vi "nano MALDI spotter v1.2.vi"() -> ()   [LabVIEW 2014]
uses:
  <vilib>/MakerHub/LINX/Public/Peripherals/Digital/Digital Write 1 Chan.vi
  <vilib>/MakerHub/LINX/Public/Peripherals/Digital/Digital Read 1 Chan.vi
  <vilib>/MakerHub/LINX/Public/Peripherals/Digital/Digital Write N Chans.vi
  <vilib>/MakerHub/LINX/Public/Peripherals/Digital/Digital Read N Chans.vi
  <vilib>/MakerHub/LINX/Private/Local IO/LinxDigitalWrite.vi
  <vilib>/MakerHub/LINX/Public/Utilities/Check Channel.vi
  <vilib>/MakerHub/LINX/Private/Local IO/LinxDigitalRead.vi
  <vilib>/MakerHub/LINX/Public/Utilities/Open Serial.vi
  <vilib>/MakerHub/LINX/Private/Utilties/Generate Error.vi
  <vilib>/MakerHub/LINX/LMH-LINX.lvlib
panel:
  out "number of spots":i8
  out "R of B/49":dbl
  out "IQ of B/49":dbl
  out "B-25":dbl
  out "First point(row)=Last point(row) ?":bool
  out "B\n=Number of spots except the first row":dbl
  out "B-1\n= # of spots in the last row\n= (# of spots - first row -1)":dbl
  out "IQ of B/25 = 0":bool
  out "IQ of B/49 = 0":bool
  out "A\n= 24-start point(column)+1\n= # of spots in the first row":dbl
  out "24-start point(columm)":dbl
  out "Last point(column)-Start point(column)":dbl
  out "milliseconds to wait 2":u32
  in  "stop":bool
  in  "Tab Control":T1(tab)=enum."Motor control"
  in  "Loop Control":bool=TRUE
  in  "Serial Port":refnum<visa-resource-name>="COM8" caption="Serial Port 2"
  in  "Digital Output Channel Channel":u8=13
  in  "LED Control":bool
  in  "OPTIONS":enum16{"OFF", "syringe", "X axis", "Y axis"}(ring)
  in  "*  Light On - Counterclockwise\n*  Light Off - Clockwise":bool
  in  "Value":bool
  in  "Value 2":bool=TRUE
  in  "FREQUENCY (Hz)":u32=50
  in  "Frequency (Hz) 2":u32(slide)=450 scale=50.0..450.0
  in  "Frequency (Hz) 3":u32(slide)=450 scale=50.0..450.0
  in  "MILLISECONDS":u32=40
  in  "SWITCH":bool=TRUE
  in  "Time per spots(s)":i8
  in  "Last point(column)":dbl
  in  "Start point(column)":dbl
  in  "Start point, row":dbl
  in  "Last point, row":dbl
  in  "RUN":bool
  in  "Total elution time\n(min)":sgl
  # "Nano-LC MALDI Spotter Robot"
  # "Instructions:\n1.Set Arduino Serial port.\n2.Choose the default LED DO channel(13). \n3.Confirm that LED control operates normally."
  # "Instructions:\n1.Change the options before operating motors\n2.Turn on the light to rotate moter counterclockwise.\n3.To speed up the motor speed, increase the FREQEUNCY and decrease MILLISECONDS.\n4.Before changing to another tab, click stop button."
  # "Instructions:\nTo start autohome, click SWITCH"
  # "Instructions:\n1. Fill in the blank. Refer to the picture below\n2. You can choose whether matrix motor will be operated or not\n3. Click RUN to start spotting"
  # "Please insert corresponding number in  \"Row\" blank box.\nA=1, B=2, C=3, D=4, E=5, F=6, G=7, H=8, I=9, J=10, K=11, \nL= 12, M=13, N=14, O=15, P=16"
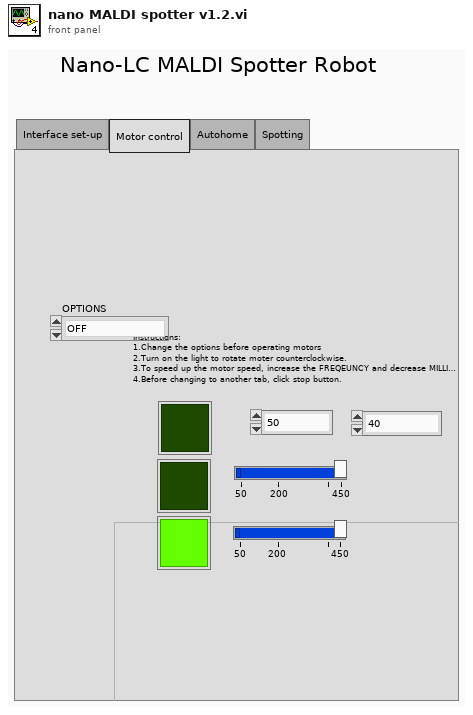
[diagram p1: front panel]
types:
  T1 = enum32{"Interface set-up", "Motor control", "Autohome", "Spotting"}
  T2 = typedef "LMH-LINX.lvlib/LINX Ref.ctl" = cluster{"IO":T3, "Interface":T4, "LINX Device Config":T5}
  T3 = typedef "LMH-LINX.lvlib/Platform.ctl" = enum16{"Remote", "Local"}
  T4 = typedef "LMH-LINX.lvlib/Interface.ctl" = enum16{"Serial", "TCP"}
  T5 = typedef "LMH-LINX.lvlib/Device.lvlib/LINX Device Config.ctl" = cluster{"Interface":T4, "COM Port":refnum<visa-resource-name>, "TCP Configuration":T6, "Device Family":u8, "Device ID":u8, "Device Name":string, "TCP Ref":refnum<k5>, "Channels":T7}
  T6 = typedef "LMH-LINX.lvlib/Device.lvlib/TCP Config.ctl" = cluster{"IP Address":string, "Port":u16}
  T7 = typedef "LMH-LINX.lvlib/Channels.ctl" = cluster{"DI":u8[], "DO":u8[], "AI":u8[], "AO":u8[], "PWM":u8[], "QE":u8[], "UART":u8[], "I2C 2":u8[], "SPI":u8[], "CAN":u8[], "Servo":u8[], "AI Ref (V)":dbl, "AI Resolution (Bits)":u8, "AO Ref (V)":dbl, "AO Resolution (Bits)":u8}
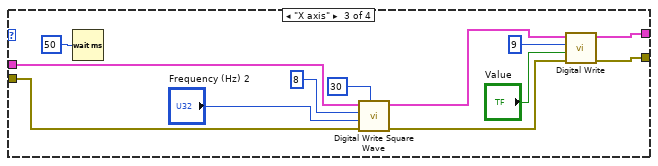
[diagram p5: hidden frame]
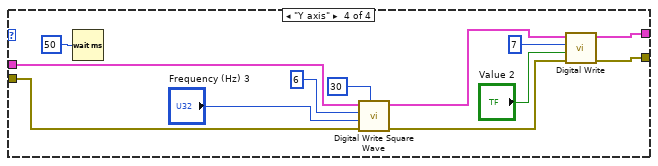
[diagram p6: hidden frame]
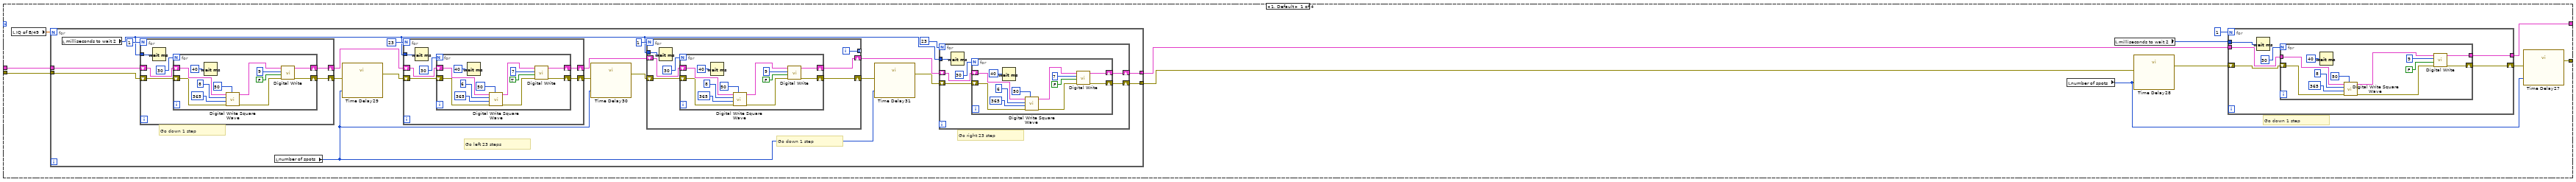
[diagram p10: hidden frame]
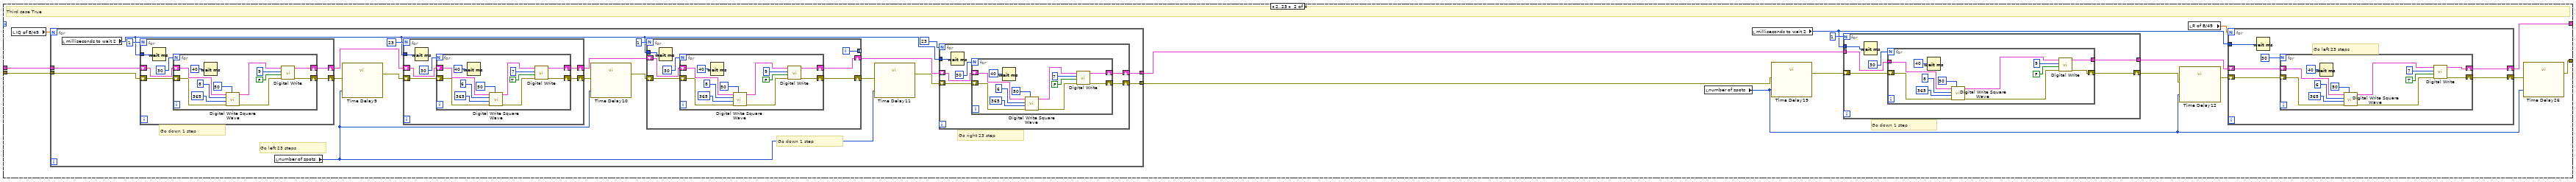
[diagram p11: hidden frame]
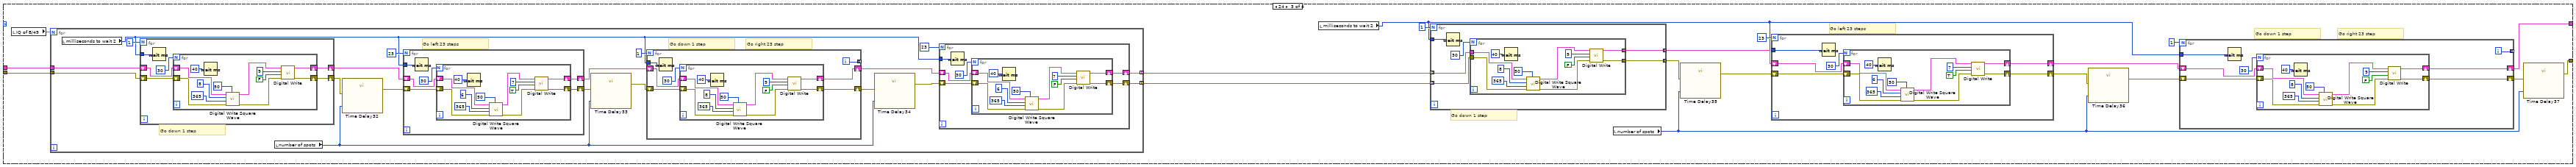
[diagram p12: hidden frame]
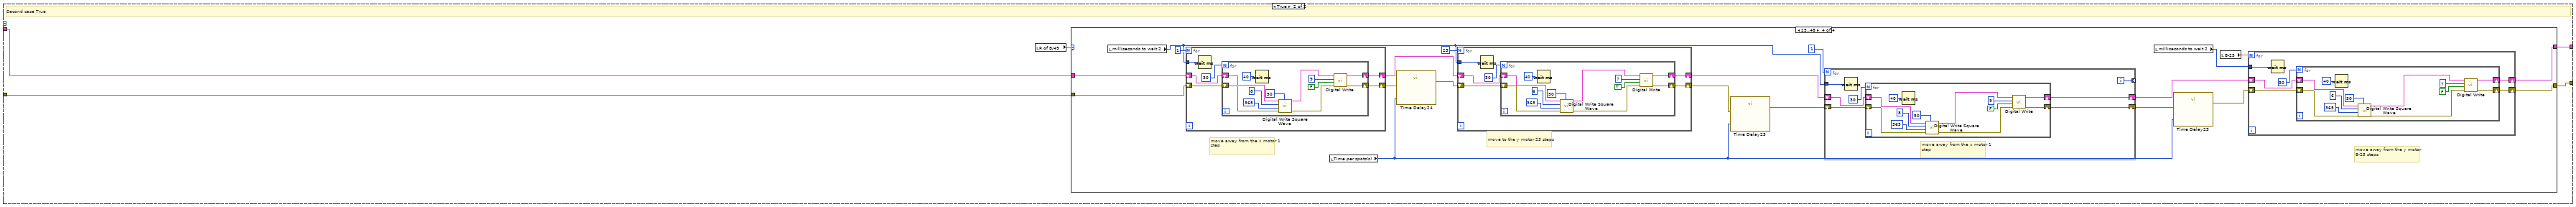
[diagram p13: hidden frame]
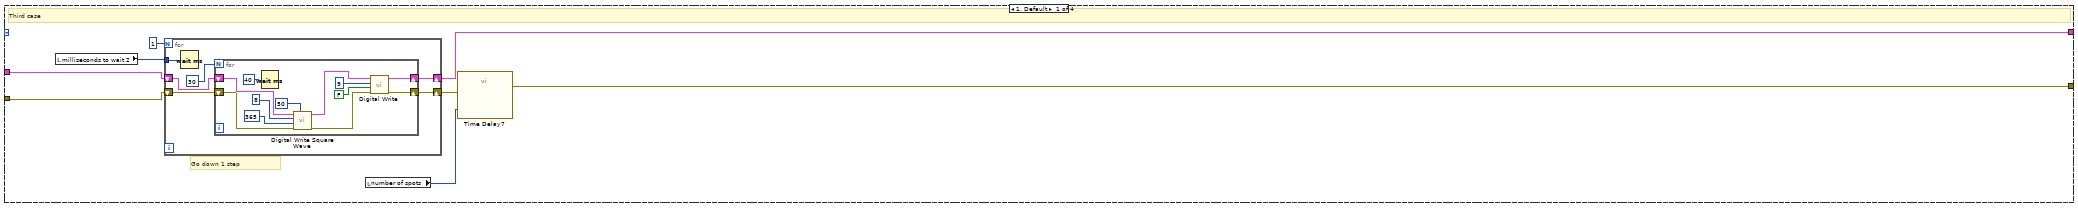
[diagram p14: hidden frame]
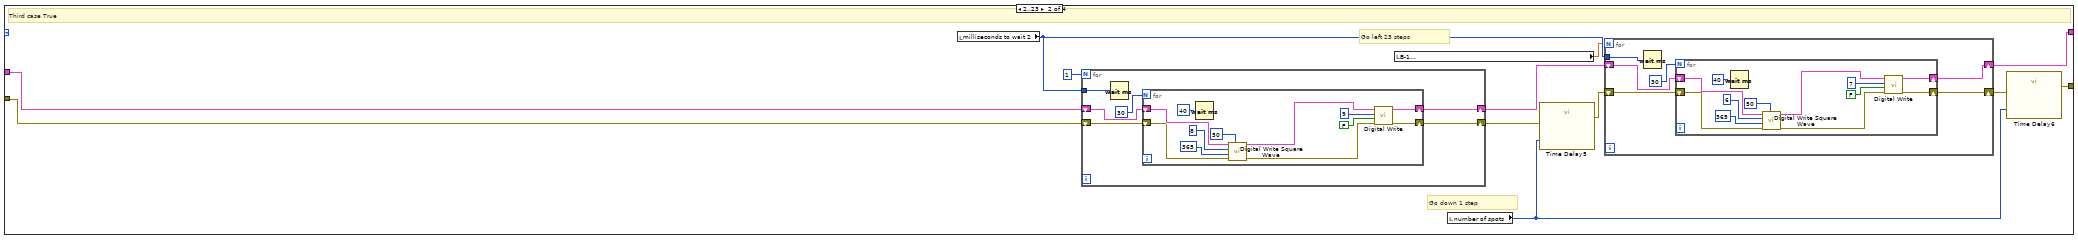
[diagram p15: hidden frame]
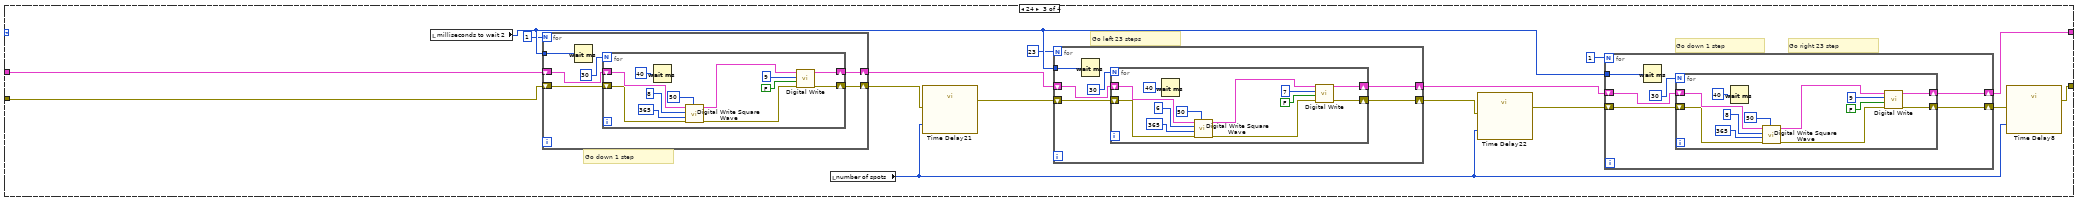
[diagram p16: hidden frame]
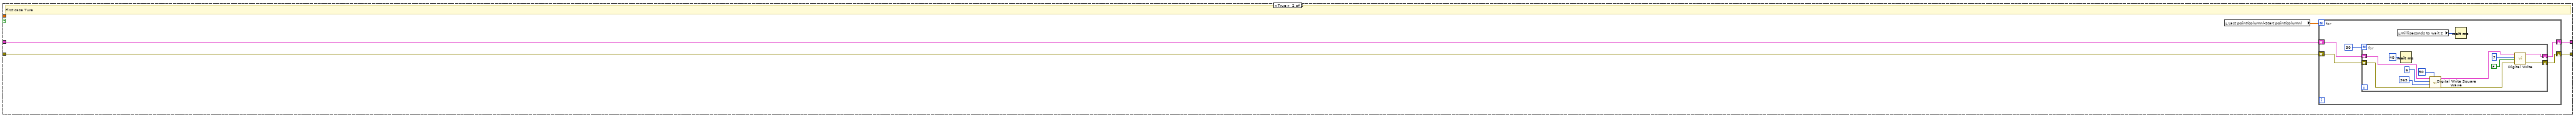
[diagram p17: hidden frame]
diagram:
  # "Option 선택용 Tab control\n-setting\n-autohome\n-motor control\n-spotting"
  # "4."
  n1 = call-poly <vilib>:"Open.vi"("Error In"=errorcluster {"status"=FALSE, "code"=0, "source"=""}, "Serial Port"="Serial Port") -> ("Error Out"=w3:errorcluster, "LINX Resource"=w4:T2)  [unwired: 7 in, 1 out]
  n2 = while {
    tunnel: w4 -> [w12]
    tunnel: w3 -> [w11]
    tunnel: [w10] -> w2
    tunnel: [w9] -> w1
    stop <- "stop" stop-if-true
    n3 = case shown="\"Spotting\"" "Tab Control" {
      tunnel: w12 -> [w17 w30 w71 w205]
      tunnel: w11 -> [w16 w29 w72 w206]
      tunnel: [w15 w28 w70 w180] -> w10
      tunnel: [w14 w27 w69 w179] -> w9
      frame "Interface set-up", Default {
        # "1. Open a connection to the LINX device.\n3. Write the value to the specified DO channel.\n4. Close the connection to the LINX device.\n5. Handle Errors"
        # "LED control\nIf it is well operated, labview and arduino is connected."
        n4 = while {
          tunnel: w17 -> [w24]
          tunnel: [w23] -> w15
          shift-right: [w21] -> w14
          shift-left: w16 -> [w22]
          stop <- w25 stop-if-true
          n5 = call-poly <vilib>:"Digital Write.vi"("Error In"=w22, "Output Value"="LED Control", "DO Channel"="Digital Output Channel Channel", "LINX Resource"=w24) -> ("Error Out"=w21:errorcluster, "LINX Resource"=w23:T2)  [unwired: 6 in]
          n6 = Or(x=w21, y="Loop Control") -> (x .or. y?=w25:bool)
        }
      }
      frame "Motor control" {
        n7 = case shown="\"syringe\"" "OPTIONS" {
          tunnel: w30 -> [w32 w44 w54 w68]
          tunnel: w29 -> [w31 w43 w53 w67]
          tunnel: [w32 w42 w56 w66] -> w28
          tunnel: [w31 w41 w55 w65] -> w27
          frame "OFF", Default {
          }
          frame "syringe" {
            # "Syringe motor On/Off\n-True=On\n-False=Off, 다른 option 대기"
            n8 = Wait (ms)(milliseconds to wait="MILLISECONDS") -> ()  [unwired: 1 out]
            n9 = call <vilib>:"Digital Write Square Wave.vi"("Duration (ms)"=u32 50, "Error In"=w43, "Frequency (Hz)"="FREQUENCY (Hz)", "Channel"=u8 10, "LINX Resource"=w44) -> ("Error Out"=w39:errorcluster, "LINX Resource"=w40:T2)  [unwired: 5 in]
            n10 = call-poly <vilib>:"Digital Write.vi"("Error In"=w39, "Output Value"="*  Light On - Counterclockwise\n*  Light Off - Clockwise", "DO Channel"=u8 11, "LINX Resource"=w40) -> ("Error Out"=w41:errorcluster, "LINX Resource"=w42:T2)  [unwired: 6 in]
          }
          frame "X axis" {
            n11 = Wait (ms)(milliseconds to wait=u32 50) -> ()  [unwired: 1 out]
            n12 = call <vilib>:"Digital Write Square Wave.vi"("Duration (ms)"=u32 30, "Error In"=w53, "Frequency (Hz)"="Frequency (Hz) 2", "Channel"=u8 8, "LINX Resource"=w54) -> ("Error Out"=w51:errorcluster, "LINX Resource"=w52:T2)  [unwired: 5 in]
            n13 = call-poly <vilib>:"Digital Write.vi"("Error In"=w51, "Output Value"="Value", "DO Channel"=u8 9, "LINX Resource"=w52) -> ("Error Out"=w55:errorcluster, "LINX Resource"=w56:T2)  [unwired: 6 in]
          }
          frame "Y axis" {
            n14 = Wait (ms)(milliseconds to wait=u32 50) -> ()  [unwired: 1 out]
            n15 = call <vilib>:"Digital Write Square Wave.vi"("Duration (ms)"=u32 30, "Error In"=w67, "Frequency (Hz)"="Frequency (Hz) 3", "Channel"=u8 6, "LINX Resource"=w68) -> ("Error Out"=w63:errorcluster, "LINX Resource"=w64:T2)  [unwired: 5 in]
            n16 = call-poly <vilib>:"Digital Write.vi"("Error In"=w63, "Output Value"="Value 2", "DO Channel"=u8 7, "LINX Resource"=w64) -> ("Error Out"=w65:errorcluster, "LINX Resource"=w66:T2)  [unwired: 6 in]
          }
        }
      }
      frame "Autohome" {
        n17 = event shown="[0] \"SWITCH\": Value Change" {
          selector: _ -> [_]
          dyn-events: _ -> [_]
          timeout: _ -> [_]
          tunnel: w72 -> [w79]
          tunnel: w71 -> [w80]
          tunnel: [w84] -> w70
          tunnel: [w83] -> w69
          event "SWITCH": Value Change {
            # "Autohome option On/Off 컨트롤"
            # "*Y axis autohome\n1) if digital reads #4, motor stops to rotate.\n2) Motor rotates to go to the position of sink."
            # "*X axis autohome\n1) if digital reads #5, motor stops to rotate.\n2) Motor rotates to go to the position of sink."
            n18 = event-data() -> ()  [unwired: 1 in, 6 out]
            n19 = while {
              tunnel: w80 -> [w108]
              tunnel: [w118] -> w78
              tunnel: [w115] -> w77
              tunnel: w79 -> [w107]
              stop <- w114 stop-if-true
              n20 = Wait (ms)(milliseconds to wait=u32 50) -> ()  [unwired: 1 out]
              n21 = call <vilib>:"Digital Write Square Wave.vi"("Duration (ms)"=u32 30, "Error In"=w107, "Frequency (Hz)"=u32 450, "Channel"=u8 8, "LINX Resource"=w108) -> ("Error Out"=w112:errorcluster, "LINX Resource"=w113:T2)  [unwired: 5 in]
              n22 = call-poly <vilib>:"Digital Write.vi"("Error In"=w112, "Output Value"=TRUE, "DO Channel"=u8 9, "LINX Resource"=w113) -> ("Error Out"=w105:errorcluster, "LINX Resource"=w106:T2)  [unwired: 6 in]
              n23 = call-poly <vilib>:"Digital Read.vi"("Error In"=w105, "DI Channel"=u8 5 ("Analog Channel"), "LINX Resource"=w106) -> ("Error Out"=w115:errorcluster, "DI Value"=w116:bool, "LINX Resource"=w118:T2)  [unwired: 6 in]
              n24 = Or(x=w116, y=w115) -> (x .or. y?=w114:bool)
            }
            n25 = for {
              N: 83 -> [_]
              tunnel: w78 -> [w135]
              tunnel: [w133] -> w76
              tunnel: [w132] -> w75
              tunnel: w77 -> [w134]
              n26 = Wait (ms)(milliseconds to wait=u32 50) -> ()  [unwired: 1 out]
              n27 = call <vilib>:"Digital Write Square Wave.vi"("Duration (ms)"=u32 50, "Error In"=w134, "Frequency (Hz)"=u32 400, "Channel"=u8 8, "LINX Resource"=w135) -> ("Error Out"=w141:errorcluster, "LINX Resource"=w142:T2)  [unwired: 5 in]
              n28 = call-poly <vilib>:"Digital Write.vi"("Error In"=w141, "Output Value"=FALSE, "DO Channel"=u8 9, "LINX Resource"=w142) -> ("Error Out"=w132:errorcluster, "LINX Resource"=w133:T2)  [unwired: 6 in]
            }
            n29 = while {
              tunnel: w76 -> [w91]
              tunnel: [w101] -> w74
              tunnel: [w98] -> w73
              tunnel: w75 -> [w90]
              stop <- w97 stop-if-true
              n30 = Wait (ms)(milliseconds to wait=u32 50) -> ()  [unwired: 1 out]
              n31 = call <vilib>:"Digital Write Square Wave.vi"("Duration (ms)"=u32 30, "Error In"=w90, "Frequency (Hz)"=u32 450, "Channel"=u8 6, "LINX Resource"=w91) -> ("Error Out"=w95:errorcluster, "LINX Resource"=w96:T2)  [unwired: 5 in]
              n32 = call-poly <vilib>:"Digital Write.vi"("Error In"=w95, "Output Value"=TRUE, "DO Channel"=u8 7, "LINX Resource"=w96) -> ("Error Out"=w88:errorcluster, "LINX Resource"=w89:T2)  [unwired: 6 in]
              n33 = call-poly <vilib>:"Digital Read.vi"("Error In"=w88, "DI Channel"=u8 4 ("Analog Channel"), "LINX Resource"=w89) -> ("Error Out"=w98:errorcluster, "DI Value"=w99:bool, "LINX Resource"=w101:T2)  [unwired: 6 in]
              n34 = Or(x=w99, y=w98) -> (x .or. y?=w97:bool)
            }
            n35 = for {
              N: 260 -> [_]
              tunnel: [w121] -> w84
              shift-right: [w120] -> w83
              shift-left: w73 -> [w130]
              tunnel: w74 -> [w122]
              n36 = Wait (ms)(milliseconds to wait=u32 50) -> ()  [unwired: 1 out]
              n37 = call <vilib>:"Digital Write Square Wave.vi"("Duration (ms)"=u32 50, "Error In"=w130, "Frequency (Hz)"=u32 400, "Channel"=u8 6, "LINX Resource"=w122) -> ("Error Out"=w128:errorcluster, "LINX Resource"=w129:T2)  [unwired: 5 in]
              n38 = call-poly <vilib>:"Digital Write.vi"("Error In"=w128, "Output Value"=FALSE, "DO Channel"=u8 7, "LINX Resource"=w129) -> ("Error Out"=w120:errorcluster, "LINX Resource"=w121:T2)  [unwired: 6 in]
            }
          }
        }
      }
      frame "Spotting" {
        # "Case 1 : Is it Row of start position=Row of last position?\nTrue : Move just as the value(Column position of last - column position of first)\nFalse :  First, move right just as the value, 24 - Start position(column)"
        # "Setting start position of row from (1,1)\nTrue : Row position of start point - 1 = 0, don't move \nFalse : Riw position of start point -1 is not 0. \n          move downward just as many as the value"
        # "Move from the position of sink to (1,1)"
        # "Setting start position of column from (1,1)\nTrue : Column position of start point - 1 = 0, don't move \nFalse : Column position of start point -1 is not 0. \n          move downward just as many as the value"
        n39 = event shown="[0] \"RUN\": Value Change" {
          selector: _ -> [_]
          dyn-events: _ -> [_]
          timeout: _ -> [_]
          tunnel: [w332] -> w209
          tunnel: [w331] -> w208
          tunnel: w206 -> [w330]
          tunnel: w205 -> [w329]
          event "RUN": Value Change {
            n40 = event-data() -> ()  [unwired: 1 in, 6 out]
            n41 = for {
              N: 130 -> [_]
              tunnel: [w354] -> w326
              shift-right: [w348] -> w325
              shift-left: w330 -> [w356]
              tunnel: w329 -> [w346]
              n42 = Wait (ms)(milliseconds to wait=u32 50) -> ()  [unwired: 1 out]
              n43 = call <vilib>:"Digital Write Square Wave.vi"("Duration (ms)"=u32 50, "Error In"=w356, "Frequency (Hz)"=u32 400, "Channel"=u8 8, "LINX Resource"=w346) -> ("Error Out"=w353:errorcluster, "LINX Resource"=w355:T2)  [unwired: 5 in]
              n44 = call-poly <vilib>:"Digital Write.vi"("Error In"=w353, "Output Value"=FALSE, "DO Channel"=u8 9, "LINX Resource"=w355) -> ("Error Out"=w348:errorcluster, "LINX Resource"=w354:T2)  [unwired: 6 in]
            }
            n45 = call "Time Delay"("error in (no error)"=w325, "Delay Time (s)"=1.0) -> ("error out"=w324:errorcluster)  [unwired: 9 in]
            n46 = for {
              N: 130 -> [_]
              tunnel: [w342] -> w332
              shift-right: [w336] -> w331
              shift-left: w324 -> [w344]
              tunnel: w326 -> [w334]
              n47 = Wait (ms)(milliseconds to wait=u32 50) -> ()  [unwired: 1 out]
              n48 = call <vilib>:"Digital Write Square Wave.vi"("Duration (ms)"=u32 50, "Error In"=w344, "Frequency (Hz)"=u32 400, "Channel"=u8 6, "LINX Resource"=w334) -> ("Error Out"=w341:errorcluster, "LINX Resource"=w343:T2)  [unwired: 5 in]
              n49 = call-poly <vilib>:"Digital Write.vi"("Error In"=w341, "Output Value"=FALSE, "DO Channel"=u8 7, "LINX Resource"=w343) -> ("Error Out"=w336:errorcluster, "LINX Resource"=w342:T2)  [unwired: 6 in]
            }
          }
        }
        n50 = Subtract(x="Last point(column)", y="Start point(column)") -> (x-y=→"Last point(column)-Start point(column)":dbl)
        n51 = Subtract(x="Start point(column)", y=1.0) -> (x-y=w165:dbl)
        n52 = Subtract(x=24.0, y="Start point(column)") -> (x-y=w160:dbl)
        "24-start point(columm)" <- w160
        n53 = Increment(x=w160) -> (x+1=→"A\n= 24-start point(column)+1\n= # of spots in the first row":dbl)
        n54 = Equal?(x=0.0, y=w165) -> (x = y?=w199:bool)
        n55 = case shown="False" w199 {
          tunnel: [w302 w321] -> w211
          tunnel: [w303 w322] -> w210
          tunnel: w209 -> [w301 w322]
          tunnel: w208 -> [w300 w321]
          tunnel: w165 -> [w299 _]
          frame False {
            n56 = for {
              N: w299 -> [_]
              shift-right: [w308] -> w303
              shift-left: w301 -> [w306]
              shift-right: [w307] -> w302
              shift-left: w300 -> [w305]
              n57 = for {
                N: 30 -> [_]
                tunnel: [w318] -> w308
                shift-right: [w312] -> w307
                shift-left: w305 -> [w320]
                tunnel: w306 -> [w309]
                n58 = Wait (ms)(milliseconds to wait=u32 40) -> ()  [unwired: 1 out]
                n59 = call <vilib>:"Digital Write Square Wave.vi"("Duration (ms)"=u32 50, "Error In"=w320, "Frequency (Hz)"=u32 365, "Channel"=u8 8, "LINX Resource"=w309) -> ("Error Out"=w317:errorcluster, "LINX Resource"=w319:T2)  [unwired: 5 in]
                n60 = call-poly <vilib>:"Digital Write.vi"("Error In"=w317, "Output Value"=TRUE, "DO Channel"=u8 9, "LINX Resource"=w319) -> ("Error Out"=w312:errorcluster, "LINX Resource"=w318:T2)  [unwired: 6 in]
              }
            }
          }
          frame True {
          }
        }
        n61 = Subtract(x=24.0, y="Start point, row") -> ()  [unwired: 1 out]
        n62 = Subtract(x="Last point, row", y="Start point, row") -> (x-y=w191:dbl)
        n63 = Subtract(x="Start point, row", y=1.0) -> (x-y=w164:dbl)
        n64 = call "Time Delay2"("error in (no error)"=w211, "Delay Time (s)"=1.0) -> ("error out"=w212:errorcluster)  [unwired: 9 in]
        n65 = Multiply(x=30.0, y=w164) -> ()  [unwired: 1 out]
        n66 = Equal?(x=0.0, y=w191) -> (x = y?=→"First point(row)=Last point(row) ?":bool)
        n67 = Equal?(x=0.0, y=w164) -> (x = y?=w198:bool)
        n68 = case shown="False" w198 {
          tunnel: w212 -> [w278 w297]
          tunnel: w210 -> [w279 w298]
          tunnel: [w277 w298] -> w207
          tunnel: [w276 w297] -> w193
          tunnel: w164 -> [w275 _]
          frame False {
            n69 = for {
              N: w275 -> [_]
              shift-right: [w282] -> w277
              shift-left: w279 -> [w284]
              shift-right: [w281] -> w276
              shift-left: w278 -> [w283]
              n70 = for {
                N: 30 -> [_]
                tunnel: [w294] -> w282
                shift-right: [w288] -> w281
                shift-left: w283 -> [w296]
                tunnel: w284 -> [w286]
                n71 = Wait (ms)(milliseconds to wait=u32 40) -> ()  [unwired: 1 out]
                n72 = call <vilib>:"Digital Write Square Wave.vi"("Duration (ms)"=u32 50, "Error In"=w296, "Frequency (Hz)"=u32 365, "Channel"=u8 6, "LINX Resource"=w286) -> ("Error Out"=w293:errorcluster, "LINX Resource"=w295:T2)  [unwired: 5 in]
                n73 = call-poly <vilib>:"Digital Write.vi"("Error In"=w293, "Output Value"=FALSE, "DO Channel"=u8 7, "LINX Resource"=w295) -> ("Error Out"=w288:errorcluster, "LINX Resource"=w294:T2)  [unwired: 6 in]
              }
            }
          }
          frame True {
            # "subVI\nSetting start position of y"
          }
        }
        n74 = local read "A\n= 24-start point(column)+1\n= # of spots in the first row"() -> (w158:dbl)
        n75 = Multiply(x="Total elution time\n(min)", y=sgl 60.0) -> (x*y=w145:sgl)
        n76 = Divide(x=w145, y="Time per spots(s)") -> (x/y=→"number of spots":sgl)
        n77 = local read "number of spots"() -> (w147:i8)
        n78 = local read "First point(row)=Last point(row) ?"() -> (w152:bool)
        n79 = Subtract(x=w147, y=w158) -> (x-y=w155:dbl)
        "B\n=Number of spots except the first row" <- w155
        n80 = call "Time Delay3"("error in (no error)"=w193, "Delay Time (s)"="Time per spots(s)") -> ("error out"=w192:errorcluster)  [unwired: 9 in]
        n81 = Decrement(x=w155) -> (x-1=→"B-1\n= # of spots in the last row\n= (# of spots - first row -1)":dbl)
        n82 = Multiply(x=u32 1000, y="Time per spots(s)") -> (x*y=→"milliseconds to wait 2":u32)
        n83 = Subtract(x=w155, y=25.0) -> (x-y=w167:dbl)
        n84 = Quotient & Remainder(x=w155, y=49.0) -> (x-y*floor(x/y)=w172:dbl, floor(x/y)=w166:dbl)
        "IQ of B/49" <- w166
        "R of B/49" <- w172
        n85 = case shown="False" w152 {
          tunnel: w192 -> [w366 w1256]
          tunnel: w207 -> [w367 w1257]
          tunnel: [w362 w1254] -> w178
          tunnel: [w361 w1255] -> w177
          tunnel: w167 -> [_ _]
          frame False {
            # "first row"
            # "First case False"
            n86 = local read "24-start point(columm)"() -> (w358:dbl)
            n87 = local read "milliseconds to wait 2"() -> (w359:u32)
            n88 = for {
              N: w358 -> [_]
              shift-right: [w1238] -> w364
              shift-left: w367 -> [w1240]
              shift-right: [w1237] -> w365
              shift-left: w366 -> [w1239]
              tunnel: w359 -> [w1235]
              n89 = Wait (ms)(milliseconds to wait=w1235) -> ()  [unwired: 1 out]
              n90 = for {
                N: 30 -> [_]
                tunnel: [w1250] -> w1238
                shift-right: [w1244] -> w1237
                shift-left: w1239 -> [w1252]
                tunnel: w1240 -> [w1241]
                n91 = Wait (ms)(milliseconds to wait=u32 40) -> ()  [unwired: 1 out]
                n92 = call <vilib>:"Digital Write Square Wave.vi"("Duration (ms)"=u32 50, "Error In"=w1252, "Frequency (Hz)"=u32 365, "Channel"=u8 6, "LINX Resource"=w1241) -> ("Error Out"=w1249:errorcluster, "LINX Resource"=w1251:T2)  [unwired: 5 in]
                n93 = call-poly <vilib>:"Digital Write.vi"("Error In"=w1249, "Output Value"=FALSE, "DO Channel"=u8 7, "LINX Resource"=w1251) -> ("Error Out"=w1244:errorcluster, "LINX Resource"=w1250:T2)  [unwired: 6 in]
              }
            }
            n94 = local read "Time per spots(s)"() -> (w360:i8)
            n95 = local read "IQ of B/49 = 0"() -> (w357:bool)
            n96 = call "Time Delay4"("error in (no error)"=w365, "Delay Time (s)"=w360) -> ("error out"=w363:errorcluster)  [unwired: 9 in]
            n97 = case shown="False" w357 {
              tunnel: w364 -> [w370 w997]
              tunnel: w363 -> [w369 w996]
              tunnel: [w372 w994] -> w362
              tunnel: [w371 w993] -> w361
              frame False {
                # "Second case False"
                n98 = local read "R of B/49"() -> (w368:dbl)
                n99 = case shown="25..48" w368 {
                  tunnel: [w375 w500 w641 w808] -> w372
                  tunnel: [w376 w506 w642 w811] -> w371
                  tunnel: w370 -> [w374 w496 w640 w827]
                  tunnel: w369 -> [w373 w495 w639 w826]
                  frame 1, Default {
                    # "Go down 1 step"
                    n100 = local read "IQ of B/49"() -> (w377:dbl)
                    n101 = for {
                      N: w377 -> [_]
                      tunnel: [w403] -> w383
                      tunnel: [w402] -> w380
                      tunnel: w374 -> [w386]
                      tunnel: w373 -> [w385]
                      # "Go right 23 step"
                      # "Go down 1 step"
                      # "Go left 23 steps"
                      # "Go down 1 step"
                      n102 = local read "milliseconds to wait 2"() -> (w387:u32)
                      n103 = for {
                        N: 1 -> [_]
                        shift-right: [w463] -> w397
                        shift-left: w386 -> [w462]
                        shift-right: [w464] -> w395
                        shift-left: w385 -> [w461]
                        tunnel: w387 -> [w459]
                        n104 = Wait (ms)(milliseconds to wait=w459) -> ()  [unwired: 1 out]
                        n105 = for {
                          N: 30 -> [_]
                          shift-right: [w475] -> w463
                          shift-left: w462 -> [w474]
                          shift-right: [w476] -> w464
                          shift-left: w461 -> [w473]
                          n106 = Wait (ms)(milliseconds to wait=u32 40) -> ()  [unwired: 1 out]
                          n107 = call <vilib>:"Digital Write Square Wave.vi"("Duration (ms)"=u32 50, "Error In"=w473, "Frequency (Hz)"=u32 365, "Channel"=u8 8, "LINX Resource"=w474) -> ("Error Out"=w471:errorcluster, "LINX Resource"=w472:T2)  [unwired: 5 in]
                          n108 = call-poly <vilib>:"Digital Write.vi"("Error In"=w471, "Output Value"=FALSE, "DO Channel"=u8 9, "LINX Resource"=w472) -> ("Error Out"=w476:errorcluster, "LINX Resource"=w475:T2)  [unwired: 6 in]
                        }
                      }
                      n109 = local read "number of spots"() -> (w388:i8)
                      n110 = call "Time Delay29"("error in (no error)"=w395, "Delay Time (s)"=w388) -> ("error out"=w396:errorcluster)  [unwired: 9 in]
                      n111 = for {
                        N: 23 -> [_]
                        shift-right: [w424] -> w398
                        shift-left: w396 -> [w427]
                        shift-right: [w426] -> w392
                        shift-left: w397 -> [w425]
                        tunnel: w387 -> [w423]
                        n112 = Wait (ms)(milliseconds to wait=w423) -> ()  [unwired: 1 out]
                        n113 = for {
                          N: 30 -> [_]
                          shift-right: [w436] -> w424
                          shift-left: w427 -> [w439]
                          shift-right: [w438] -> w426
                          shift-left: w425 -> [w437]
                          n114 = Wait (ms)(milliseconds to wait=u32 40) -> ()  [unwired: 1 out]
                          n115 = call <vilib>:"Digital Write Square Wave.vi"("Duration (ms)"=u32 50, "Error In"=w439, "Frequency (Hz)"=u32 365, "Channel"=u8 6, "LINX Resource"=w437) -> ("Error Out"=w434:errorcluster, "LINX Resource"=w435:T2)  [unwired: 5 in]
                          n116 = call-poly <vilib>:"Digital Write.vi"("Error In"=w434, "Output Value"=TRUE, "DO Channel"=u8 7, "LINX Resource"=w435) -> ("Error Out"=w436:errorcluster, "LINX Resource"=w438:T2)  [unwired: 6 in]
                        }
                      }
                      n117 = call "Time Delay30"("error in (no error)"=w398, "Delay Time (s)"=w388) -> ("error out"=w399:errorcluster)  [unwired: 9 in]
                      n118 = for {
                        N: 1 -> [_]
                        shift-right: [w446] -> w391
                        shift-left: w392 -> [w444]
                        shift-right: [w445] -> w400
                        shift-left: w399 -> [w443]
                        tunnel: [w441] -> _ mode=indexing
                        tunnel: w387 -> [w440]
                        i -> [w441]
                        n119 = Wait (ms)(milliseconds to wait=w440) -> ()  [unwired: 1 out]
                        n120 = for {
                          N: 30 -> [_]
                          shift-right: [w458] -> w446
                          shift-left: w444 -> [w456]
                          shift-right: [w457] -> w445
                          shift-left: w443 -> [w455]
                          n121 = Wait (ms)(milliseconds to wait=u32 40) -> ()  [unwired: 1 out]
                          n122 = call <vilib>:"Digital Write Square Wave.vi"("Duration (ms)"=u32 50, "Error In"=w455, "Frequency (Hz)"=u32 365, "Channel"=u8 8, "LINX Resource"=w456) -> ("Error Out"=w447:errorcluster, "LINX Resource"=w454:T2)  [unwired: 5 in]
                          n123 = call-poly <vilib>:"Digital Write.vi"("Error In"=w447, "Output Value"=FALSE, "DO Channel"=u8 9, "LINX Resource"=w454) -> ("Error Out"=w457:errorcluster, "LINX Resource"=w458:T2)  [unwired: 6 in]
                        }
                      }
                      n124 = call "Time Delay31"("error in (no error)"=w400, "Delay Time (s)"=w388) -> ("error out"=w390:errorcluster)  [unwired: 9 in]
                      n125 = for {
                        N: 23 -> [_]
                        shift-right: [w408] -> w403
                        shift-left: w391 -> [w409]
                        shift-right: [w406] -> w402
                        shift-left: w390 -> [w407]
                        tunnel: w387 -> [w404]
                        n126 = Wait (ms)(milliseconds to wait=w404) -> ()  [unwired: 1 out]
                        n127 = for {
                          N: 30 -> [_]
                          shift-right: [w420] -> w408
                          shift-left: w409 -> [w421]
                          shift-right: [w410] -> w406
                          shift-left: w407 -> [w419]
                          n128 = Wait (ms)(milliseconds to wait=u32 40) -> ()  [unwired: 1 out]
                          n129 = call <vilib>:"Digital Write Square Wave.vi"("Duration (ms)"=u32 50, "Error In"=w419, "Frequency (Hz)"=u32 365, "Channel"=u8 6, "LINX Resource"=w421) -> ("Error Out"=w411:errorcluster, "LINX Resource"=w418:T2)  [unwired: 5 in]
                          n130 = call-poly <vilib>:"Digital Write.vi"("Error In"=w411, "Output Value"=FALSE, "DO Channel"=u8 7, "LINX Resource"=w418) -> ("Error Out"=w410:errorcluster, "LINX Resource"=w420:T2)  [unwired: 6 in]
                        }
                      }
                    }
                    n131 = local read "number of spots"() -> (w378:i8)
                    n132 = local read "milliseconds to wait 2"() -> (w379:u32)
                    n133 = call "Time Delay28"("error in (no error)"=w380, "Delay Time (s)"=w378) -> ("error out"=w382:errorcluster)  [unwired: 9 in]
                    n134 = for {
                      N: 1 -> [_]
                      tunnel: [w482] -> w376
                      tunnel: w383 -> [w480]
                      shift-right: [w481] -> w384
                      shift-left: w382 -> [w479]
                      tunnel: w379 -> [w477]
                      n135 = Wait (ms)(milliseconds to wait=w477) -> ()  [unwired: 1 out]
                      n136 = for {
                        N: 30 -> [_]
                        tunnel: [w494] -> w482
                        tunnel: w480 -> [w492]
                        shift-right: [w493] -> w481
                        shift-left: w479 -> [w491]
                        n137 = Wait (ms)(milliseconds to wait=u32 40) -> ()  [unwired: 1 out]
                        n138 = call <vilib>:"Digital Write Square Wave.vi"("Duration (ms)"=u32 50, "Error In"=w491, "Frequency (Hz)"=u32 365, "Channel"=u8 8, "LINX Resource"=w492) -> ("Error Out"=w489:errorcluster, "LINX Resource"=w490:T2)  [unwired: 5 in]
                        n139 = call-poly <vilib>:"Digital Write.vi"("Error In"=w489, "Output Value"=FALSE, "DO Channel"=u8 9, "LINX Resource"=w490) -> ("Error Out"=w493:errorcluster, "LINX Resource"=w494:T2)  [unwired: 6 in]
                      }
                    }
                    n140 = call "Time Delay27"("error in (no error)"=w384, "Delay Time (s)"=w378) -> ("error out"=w375:errorcluster)  [unwired: 9 in]
                  }
                  frame 2..23 {
                    # "Go down 1 step"
                    # "Third case True"
                    n141 = local read "IQ of B/49"() -> (w498:dbl)
                    n142 = for {
                      N: w498 -> [_]
                      tunnel: [w529] -> w507
                      tunnel: [w528] -> w503
                      tunnel: w496 -> [w512]
                      tunnel: w495 -> [w511]
                      # "Go right 23 step"
                      # "Go down 1 step"
                      # "Go left 23 steps"
                      # "Go down 1 step"
                      n143 = local read "milliseconds to wait 2"() -> (w513:u32)
                      n144 = for {
                        N: 1 -> [_]
                        shift-right: [w589] -> w523
                        shift-left: w512 -> [w588]
                        shift-right: [w590] -> w521
                        shift-left: w511 -> [w587]
                        tunnel: w513 -> [w585]
                        n145 = Wait (ms)(milliseconds to wait=w585) -> ()  [unwired: 1 out]
                        n146 = for {
                          N: 30 -> [_]
                          shift-right: [w601] -> w589
                          shift-left: w588 -> [w600]
                          shift-right: [w602] -> w590
                          shift-left: w587 -> [w599]
                          n147 = Wait (ms)(milliseconds to wait=u32 40) -> ()  [unwired: 1 out]
                          n148 = call <vilib>:"Digital Write Square Wave.vi"("Duration (ms)"=u32 50, "Error In"=w599, "Frequency (Hz)"=u32 365, "Channel"=u8 8, "LINX Resource"=w600) -> ("Error Out"=w597:errorcluster, "LINX Resource"=w598:T2)  [unwired: 5 in]
                          n149 = call-poly <vilib>:"Digital Write.vi"("Error In"=w597, "Output Value"=FALSE, "DO Channel"=u8 9, "LINX Resource"=w598) -> ("Error Out"=w602:errorcluster, "LINX Resource"=w601:T2)  [unwired: 6 in]
                        }
                      }
                      n150 = local read "number of spots"() -> (w514:i8)
                      n151 = call "Time Delay9"("error in (no error)"=w521, "Delay Time (s)"=w514) -> ("error out"=w522:errorcluster)  [unwired: 9 in]
                      n152 = for {
                        N: 23 -> [_]
                        shift-right: [w550] -> w524
                        shift-left: w522 -> [w553]
                        shift-right: [w552] -> w518
                        shift-left: w523 -> [w551]
                        tunnel: w513 -> [w549]
                        n153 = Wait (ms)(milliseconds to wait=w549) -> ()  [unwired: 1 out]
                        n154 = for {
                          N: 30 -> [_]
                          shift-right: [w562] -> w550
                          shift-left: w553 -> [w565]
                          shift-right: [w564] -> w552
                          shift-left: w551 -> [w563]
                          n155 = Wait (ms)(milliseconds to wait=u32 40) -> ()  [unwired: 1 out]
                          n156 = call <vilib>:"Digital Write Square Wave.vi"("Duration (ms)"=u32 50, "Error In"=w565, "Frequency (Hz)"=u32 365, "Channel"=u8 6, "LINX Resource"=w563) -> ("Error Out"=w560:errorcluster, "LINX Resource"=w561:T2)  [unwired: 5 in]
                          n157 = call-poly <vilib>:"Digital Write.vi"("Error In"=w560, "Output Value"=TRUE, "DO Channel"=u8 7, "LINX Resource"=w561) -> ("Error Out"=w562:errorcluster, "LINX Resource"=w564:T2)  [unwired: 6 in]
                        }
                      }
                      n158 = call "Time Delay10"("error in (no error)"=w524, "Delay Time (s)"=w514) -> ("error out"=w525:errorcluster)  [unwired: 9 in]
                      n159 = for {
                        N: 1 -> [_]
                        shift-right: [w572] -> w517
                        shift-left: w518 -> [w570]
                        shift-right: [w571] -> w526
                        shift-left: w525 -> [w569]
                        tunnel: [w567] -> _ mode=indexing
                        tunnel: w513 -> [w566]
                        i -> [w567]
                        n160 = Wait (ms)(milliseconds to wait=w566) -> ()  [unwired: 1 out]
                        n161 = for {
                          N: 30 -> [_]
                          shift-right: [w584] -> w572
                          shift-left: w570 -> [w582]
                          shift-right: [w583] -> w571
                          shift-left: w569 -> [w581]
                          n162 = Wait (ms)(milliseconds to wait=u32 40) -> ()  [unwired: 1 out]
                          n163 = call <vilib>:"Digital Write Square Wave.vi"("Duration (ms)"=u32 50, "Error In"=w581, "Frequency (Hz)"=u32 365, "Channel"=u8 8, "LINX Resource"=w582) -> ("Error Out"=w573:errorcluster, "LINX Resource"=w580:T2)  [unwired: 5 in]
                          n164 = call-poly <vilib>:"Digital Write.vi"("Error In"=w573, "Output Value"=FALSE, "DO Channel"=u8 9, "LINX Resource"=w580) -> ("Error Out"=w583:errorcluster, "LINX Resource"=w584:T2)  [unwired: 6 in]
                        }
                      }
                      n165 = call "Time Delay11"("error in (no error)"=w526, "Delay Time (s)"=w514) -> ("error out"=w516:errorcluster)  [unwired: 9 in]
                      n166 = for {
                        N: 23 -> [_]
                        shift-right: [w534] -> w529
                        shift-left: w517 -> [w535]
                        shift-right: [w532] -> w528
                        shift-left: w516 -> [w533]
                        tunnel: w513 -> [w530]
                        n167 = Wait (ms)(milliseconds to wait=w530) -> ()  [unwired: 1 out]
                        n168 = for {
                          N: 30 -> [_]
                          shift-right: [w546] -> w534
                          shift-left: w535 -> [w547]
                          shift-right: [w536] -> w532
                          shift-left: w533 -> [w545]
                          n169 = Wait (ms)(milliseconds to wait=u32 40) -> ()  [unwired: 1 out]
                          n170 = call <vilib>:"Digital Write Square Wave.vi"("Duration (ms)"=u32 50, "Error In"=w545, "Frequency (Hz)"=u32 365, "Channel"=u8 6, "LINX Resource"=w547) -> ("Error Out"=w537:errorcluster, "LINX Resource"=w544:T2)  [unwired: 5 in]
                          n171 = call-poly <vilib>:"Digital Write.vi"("Error In"=w537, "Output Value"=FALSE, "DO Channel"=u8 7, "LINX Resource"=w544) -> ("Error Out"=w536:errorcluster, "LINX Resource"=w546:T2)  [unwired: 6 in]
                        }
                      }
                    }
                    n172 = local read "number of spots"() -> (w499:i8)
                    n173 = local read "milliseconds to wait 2"() -> (w502:u32)
                    n174 = call "Time Delay19"("error in (no error)"=w503, "Delay Time (s)"=w499) -> ("error out"=w505:errorcluster)  [unwired: 9 in]
                    n175 = for {
                      N: 1 -> [_]
                      tunnel: [w626] -> w510
                      tunnel: w507 -> [w624]
                      shift-right: [w625] -> w508
                      shift-left: w505 -> [w623]
                      tunnel: w502 -> [w621]
                      n176 = Wait (ms)(milliseconds to wait=w621) -> ()  [unwired: 1 out]
                      n177 = for {
                        N: 30 -> [_]
                        tunnel: [w638] -> w626
                        tunnel: w624 -> [w636]
                        shift-right: [w637] -> w625
                        shift-left: w623 -> [w635]
                        n178 = Wait (ms)(milliseconds to wait=u32 40) -> ()  [unwired: 1 out]
                        n179 = call <vilib>:"Digital Write Square Wave.vi"("Duration (ms)"=u32 50, "Error In"=w635, "Frequency (Hz)"=u32 365, "Channel"=u8 8, "LINX Resource"=w636) -> ("Error Out"=w633:errorcluster, "LINX Resource"=w634:T2)  [unwired: 5 in]
                        n180 = call-poly <vilib>:"Digital Write.vi"("Error In"=w633, "Output Value"=FALSE, "DO Channel"=u8 9, "LINX Resource"=w634) -> ("Error Out"=w637:errorcluster, "LINX Resource"=w638:T2)  [unwired: 6 in]
                      }
                    }
                    n181 = call "Time Delay12"("error in (no error)"=w508, "Delay Time (s)"=w499) -> ("error out"=w509:errorcluster)  [unwired: 9 in]
                    n182 = local read "R of B/49"() -> (w497:dbl)
                    n183 = for {
                      N: w497 -> [_]
                      shift-right: [w605] -> w506
                      shift-left: w510 -> [w608]
                      shift-right: [w606] -> w501
                      shift-left: w509 -> [w607]
                      tunnel: w502 -> [w604]
                      # "Go left 23 steps"
                      n184 = Wait (ms)(milliseconds to wait=w604) -> ()  [unwired: 1 out]
                      n185 = for {
                        N: 30 -> [_]
                        shift-right: [w617] -> w606
                        shift-left: w607 -> [w620]
                        shift-right: [w619] -> w605
                        shift-left: w608 -> [w618]
                        n186 = Wait (ms)(milliseconds to wait=u32 40) -> ()  [unwired: 1 out]
                        n187 = call <vilib>:"Digital Write Square Wave.vi"("Duration (ms)"=u32 50, "Error In"=w620, "Frequency (Hz)"=u32 365, "Channel"=u8 6, "LINX Resource"=w618) -> ("Error Out"=w615:errorcluster, "LINX Resource"=w616:T2)  [unwired: 5 in]
                        n188 = call-poly <vilib>:"Digital Write.vi"("Error In"=w615, "Output Value"=TRUE, "DO Channel"=u8 7, "LINX Resource"=w616) -> ("Error Out"=w617:errorcluster, "LINX Resource"=w619:T2)  [unwired: 6 in]
                      }
                    }
                    n189 = call "Time Delay26"("error in (no error)"=w501, "Delay Time (s)"=w499) -> ("error out"=w500:errorcluster)  [unwired: 9 in]
                  }
                  frame 24 {
                    # "Go right 23 step"
                    # "Go down 1 step"
                    # "Go left 23 steps"
                    # "Go down 1 step"
                    n190 = local read "IQ of B/49"() -> (w643:dbl)
                    n191 = for {
                      N: w643 -> [_]
                      tunnel: [w719] -> w648 mode=indexing
                      tunnel: [w718] -> w647 mode=indexing
                      tunnel: w640 -> [w716]
                      tunnel: w639 -> [w715]
                      # "Go right 23 step"
                      # "Go down 1 step"
                      # "Go left 23 steps"
                      # "Go down 1 step"
                      n192 = local read "milliseconds to wait 2"() -> (w713:u32)
                      n193 = for {
                        N: 1 -> [_]
                        shift-right: [w773] -> w726
                        shift-left: w716 -> [w772]
                        shift-right: [w774] -> w724
                        shift-left: w715 -> [w771]
                        tunnel: w713 -> [w769]
                        n194 = Wait (ms)(milliseconds to wait=w769) -> ()  [unwired: 1 out]
                        n195 = for {
                          N: 30 -> [_]
                          shift-right: [w785] -> w773
                          shift-left: w772 -> [w784]
                          shift-right: [w786] -> w774
                          shift-left: w771 -> [w783]
                          n196 = Wait (ms)(milliseconds to wait=u32 40) -> ()  [unwired: 1 out]
                          n197 = call <vilib>:"Digital Write Square Wave.vi"("Duration (ms)"=u32 50, "Error In"=w783, "Frequency (Hz)"=u32 365, "Channel"=u8 8, "LINX Resource"=w784) -> ("Error Out"=w781:errorcluster, "LINX Resource"=w782:T2)  [unwired: 5 in]
                          n198 = call-poly <vilib>:"Digital Write.vi"("Error In"=w781, "Output Value"=FALSE, "DO Channel"=u8 9, "LINX Resource"=w782) -> ("Error Out"=w786:errorcluster, "LINX Resource"=w785:T2)  [unwired: 6 in]
                        }
                      }
                      n199 = local read "number of spots"() -> (w714:i8)
                      n200 = call "Time Delay32"("error in (no error)"=w724, "Delay Time (s)"=w714) -> ("error out"=w725:errorcluster)  [unwired: 9 in]
                      n201 = for {
                        N: 23 -> [_]
                        shift-right: [w734] -> w727
                        shift-left: w725 -> [w737]
                        shift-right: [w736] -> w721
                        shift-left: w726 -> [w735]
                        tunnel: w713 -> [w733]
                        n202 = Wait (ms)(milliseconds to wait=w733) -> ()  [unwired: 1 out]
                        n203 = for {
                          N: 30 -> [_]
                          shift-right: [w746] -> w734
                          shift-left: w737 -> [w749]
                          shift-right: [w748] -> w736
                          shift-left: w735 -> [w747]
                          n204 = Wait (ms)(milliseconds to wait=u32 40) -> ()  [unwired: 1 out]
                          n205 = call <vilib>:"Digital Write Square Wave.vi"("Duration (ms)"=u32 50, "Error In"=w749, "Frequency (Hz)"=u32 365, "Channel"=u8 6, "LINX Resource"=w747) -> ("Error Out"=w744:errorcluster, "LINX Resource"=w745:T2)  [unwired: 5 in]
                          n206 = call-poly <vilib>:"Digital Write.vi"("Error In"=w744, "Output Value"=TRUE, "DO Channel"=u8 7, "LINX Resource"=w745) -> ("Error Out"=w746:errorcluster, "LINX Resource"=w748:T2)  [unwired: 6 in]
                        }
                      }
                      n207 = call "Time Delay33"("error in (no error)"=w727, "Delay Time (s)"=w714) -> ("error out"=w728:errorcluster)  [unwired: 9 in]
                      n208 = for {
                        N: 1 -> [_]
                        shift-right: [w756] -> w720
                        shift-left: w721 -> [w754]
                        shift-right: [w755] -> w730
                        shift-left: w728 -> [w753]
                        tunnel: [w751] -> _ mode=indexing
                        tunnel: w713 -> [w750]
                        i -> [w751]
                        n209 = Wait (ms)(milliseconds to wait=w750) -> ()  [unwired: 1 out]
                        n210 = for {
                          N: 30 -> [_]
                          shift-right: [w768] -> w756
                          shift-left: w754 -> [w766]
                          shift-right: [w767] -> w755
                          shift-left: w753 -> [w765]
                          n211 = Wait (ms)(milliseconds to wait=u32 40) -> ()  [unwired: 1 out]
                          n212 = call <vilib>:"Digital Write Square Wave.vi"("Duration (ms)"=u32 50, "Error In"=w765, "Frequency (Hz)"=u32 365, "Channel"=u8 8, "LINX Resource"=w766) -> ("Error Out"=w757:errorcluster, "LINX Resource"=w764:T2)  [unwired: 5 in]
                          n213 = call-poly <vilib>:"Digital Write.vi"("Error In"=w757, "Output Value"=FALSE, "DO Channel"=u8 9, "LINX Resource"=w764) -> ("Error Out"=w767:errorcluster, "LINX Resource"=w768:T2)  [unwired: 6 in]
                        }
                      }
                      n214 = call "Time Delay34"("error in (no error)"=w730, "Delay Time (s)"=w714) -> ("error out"=w729:errorcluster)  [unwired: 9 in]
                      n215 = for {
                        N: 23 -> [_]
                        shift-right: [w789] -> w718
                        shift-left: w720 -> [w792]
                        shift-right: [w790] -> w719
                        shift-left: w729 -> [w791]
                        tunnel: w713 -> [w787]
                        n216 = Wait (ms)(milliseconds to wait=w787) -> ()  [unwired: 1 out]
                        n217 = for {
                          N: 30 -> [_]
                          shift-right: [w801] -> w789
                          shift-left: w792 -> [w804]
                          shift-right: [w802] -> w790
                          shift-left: w791 -> [w803]
                          n218 = Wait (ms)(milliseconds to wait=u32 40) -> ()  [unwired: 1 out]
                          n219 = call <vilib>:"Digital Write Square Wave.vi"("Duration (ms)"=u32 50, "Error In"=w803, "Frequency (Hz)"=u32 365, "Channel"=u8 6, "LINX Resource"=w804) -> ("Error Out"=w793:errorcluster, "LINX Resource"=w800:T2)  [unwired: 5 in]
                          n220 = call-poly <vilib>:"Digital Write.vi"("Error In"=w793, "Output Value"=FALSE, "DO Channel"=u8 7, "LINX Resource"=w800) -> ("Error Out"=w802:errorcluster, "LINX Resource"=w801:T2)  [unwired: 6 in]
                        }
                      }
                    }
                    n221 = local read "milliseconds to wait 2"() -> (w645:u32)
                    n222 = for {
                      N: 1 -> [_]
                      tunnel: [w663] -> w653
                      tunnel: [w662] -> w651
                      tunnel: w648 -> [w661] mode=indexing
                      tunnel: w647 -> [w660] mode=indexing
                      tunnel: w645 -> [w659]
                      n223 = Wait (ms)(milliseconds to wait=w659) -> ()  [unwired: 1 out]
                      n224 = for {
                        N: 30 -> [_]
                        tunnel: [w675] -> w663
                        tunnel: [w674] -> w662
                        tunnel: w661 -> [w673]
                        tunnel: w660 -> [w672]
                        n225 = Wait (ms)(milliseconds to wait=u32 40) -> ()  [unwired: 1 out]
                        n226 = call <vilib>:"Digital Write Square Wave.vi"("Duration (ms)"=u32 50, "Error In"=w673, "Frequency (Hz)"=u32 365, "Channel"=u8 8, "LINX Resource"=w672) -> ("Error Out"=w670:errorcluster, "LINX Resource"=w671:T2)  [unwired: 5 in]
                        n227 = call-poly <vilib>:"Digital Write.vi"("Error In"=w670, "Output Value"=FALSE, "DO Channel"=u8 9, "LINX Resource"=w671) -> ("Error Out"=w674:errorcluster, "LINX Resource"=w675:T2)  [unwired: 6 in]
                      }
                    }
                    n228 = local read "number of spots"() -> (w644:i8)
                    n229 = call "Time Delay35"("error in (no error)"=w651, "Delay Time (s)"=w644) -> ("error out"=w652:errorcluster)  [unwired: 9 in]
                    n230 = for {
                      N: 23 -> [_]
                      shift-right: [w678] -> w654
                      shift-left: w652 -> [w681]
                      shift-right: [w680] -> w649
                      shift-left: w653 -> [w679]
                      tunnel: w645 -> [w677]
                      n231 = Wait (ms)(milliseconds to wait=w677) -> ()  [unwired: 1 out]
                      n232 = for {
                        N: 30 -> [_]
                        shift-right: [w690] -> w678
                        shift-left: w681 -> [w693]
                        shift-right: [w692] -> w680
                        shift-left: w679 -> [w691]
                        n233 = Wait (ms)(milliseconds to wait=u32 40) -> ()  [unwired: 1 out]
                        n234 = call <vilib>:"Digital Write Square Wave.vi"("Duration (ms)"=u32 50, "Error In"=w693, "Frequency (Hz)"=u32 365, "Channel"=u8 6, "LINX Resource"=w691) -> ("Error Out"=w688:errorcluster, "LINX Resource"=w689:T2)  [unwired: 5 in]
                        n235 = call-poly <vilib>:"Digital Write.vi"("Error In"=w688, "Output Value"=TRUE, "DO Channel"=u8 7, "LINX Resource"=w689) -> ("Error Out"=w690:errorcluster, "LINX Resource"=w692:T2)  [unwired: 6 in]
                      }
                    }
                    n236 = call "Time Delay36"("error in (no error)"=w654, "Delay Time (s)"=w644) -> ("error out"=w655:errorcluster)  [unwired: 9 in]
                    n237 = for {
                      N: 1 -> [_]
                      shift-right: [w700] -> w642
                      shift-left: w649 -> [w698]
                      shift-right: [w699] -> w656
                      shift-left: w655 -> [w697]
                      tunnel: [w695] -> _ mode=indexing
                      tunnel: w645 -> [w694]
                      i -> [w695]
                      n238 = Wait (ms)(milliseconds to wait=w694) -> ()  [unwired: 1 out]
                      n239 = for {
                        N: 30 -> [_]
                        shift-right: [w712] -> w700
                        shift-left: w698 -> [w710]
                        shift-right: [w711] -> w699
                        shift-left: w697 -> [w709]
                        n240 = Wait (ms)(milliseconds to wait=u32 40) -> ()  [unwired: 1 out]
                        n241 = call <vilib>:"Digital Write Square Wave.vi"("Duration (ms)"=u32 50, "Error In"=w709, "Frequency (Hz)"=u32 365, "Channel"=u8 8, "LINX Resource"=w710) -> ("Error Out"=w701:errorcluster, "LINX Resource"=w708:T2)  [unwired: 5 in]
                        n242 = call-poly <vilib>:"Digital Write.vi"("Error In"=w701, "Output Value"=FALSE, "DO Channel"=u8 9, "LINX Resource"=w708) -> ("Error Out"=w711:errorcluster, "LINX Resource"=w712:T2)  [unwired: 6 in]
                      }
                    }
                    n243 = call "Time Delay37"("error in (no error)"=w656, "Delay Time (s)"=w644) -> ("error out"=w641:errorcluster)  [unwired: 9 in]
                  }
                  frame 25..48 {
                    # "Go right 23 step"
                    # "Go down 1 step"
                    # "Go left 23 steps"
                    # "Go down 1 step"
                    # "Third case False, IQ>=1"
                    n244 = local read "IQ of B/49"() -> (w806:dbl)
                    n245 = for {
                      N: w806 -> [_]
                      tunnel: [w907] -> w814 mode=indexing
                      tunnel: [w906] -> w813 mode=indexing
                      tunnel: w827 -> [w904]
                      tunnel: w826 -> [w903]
                      # "Go right 23 step"
                      # "Go down 1 step"
                      # "Go left 23 steps"
                      # "Go down 1 step"
                      n246 = local read "milliseconds to wait 2"() -> (w901:u32)
                      n247 = for {
                        N: 1 -> [_]
                        shift-right: [w961] -> w914
                        shift-left: w904 -> [w960]
                        shift-right: [w962] -> w912
                        shift-left: w903 -> [w959]
                        tunnel: w901 -> [w957]
                        n248 = Wait (ms)(milliseconds to wait=w957) -> ()  [unwired: 1 out]
                        n249 = for {
                          N: 30 -> [_]
                          shift-right: [w973] -> w961
                          shift-left: w960 -> [w972]
                          shift-right: [w974] -> w962
                          shift-left: w959 -> [w971]
                          n250 = Wait (ms)(milliseconds to wait=u32 40) -> ()  [unwired: 1 out]
                          n251 = call <vilib>:"Digital Write Square Wave.vi"("Duration (ms)"=u32 50, "Error In"=w971, "Frequency (Hz)"=u32 365, "Channel"=u8 8, "LINX Resource"=w972) -> ("Error Out"=w969:errorcluster, "LINX Resource"=w970:T2)  [unwired: 5 in]
                          n252 = call-poly <vilib>:"Digital Write.vi"("Error In"=w969, "Output Value"=FALSE, "DO Channel"=u8 9, "LINX Resource"=w970) -> ("Error Out"=w974:errorcluster, "LINX Resource"=w973:T2)  [unwired: 6 in]
                        }
                      }
                      n253 = local read "number of spots"() -> (w902:i8)
                      n254 = call "Time Delay13"("error in (no error)"=w912, "Delay Time (s)"=w902) -> ("error out"=w913:errorcluster)  [unwired: 9 in]
                      n255 = for {
                        N: 23 -> [_]
                        shift-right: [w922] -> w915
                        shift-left: w913 -> [w925]
                        shift-right: [w924] -> w909
                        shift-left: w914 -> [w923]
                        tunnel: w901 -> [w921]
                        n256 = Wait (ms)(milliseconds to wait=w921) -> ()  [unwired: 1 out]
                        n257 = for {
                          N: 30 -> [_]
                          shift-right: [w934] -> w922
                          shift-left: w925 -> [w937]
                          shift-right: [w936] -> w924
                          shift-left: w923 -> [w935]
                          n258 = Wait (ms)(milliseconds to wait=u32 40) -> ()  [unwired: 1 out]
                          n259 = call <vilib>:"Digital Write Square Wave.vi"("Duration (ms)"=u32 50, "Error In"=w937, "Frequency (Hz)"=u32 365, "Channel"=u8 6, "LINX Resource"=w935) -> ("Error Out"=w932:errorcluster, "LINX Resource"=w933:T2)  [unwired: 5 in]
                          n260 = call-poly <vilib>:"Digital Write.vi"("Error In"=w932, "Output Value"=TRUE, "DO Channel"=u8 7, "LINX Resource"=w933) -> ("Error Out"=w934:errorcluster, "LINX Resource"=w936:T2)  [unwired: 6 in]
                        }
                      }
                      n261 = call "Time Delay14"("error in (no error)"=w915, "Delay Time (s)"=w902) -> ("error out"=w916:errorcluster)  [unwired: 9 in]
                      n262 = for {
                        N: 1 -> [_]
                        shift-right: [w944] -> w908
                        shift-left: w909 -> [w942]
                        shift-right: [w943] -> w918
                        shift-left: w916 -> [w941]
                        tunnel: [w939] -> _ mode=indexing
                        tunnel: w901 -> [w938]
                        i -> [w939]
                        n263 = Wait (ms)(milliseconds to wait=w938) -> ()  [unwired: 1 out]
                        n264 = for {
                          N: 30 -> [_]
                          shift-right: [w956] -> w944
                          shift-left: w942 -> [w954]
                          shift-right: [w955] -> w943
                          shift-left: w941 -> [w953]
                          n265 = Wait (ms)(milliseconds to wait=u32 40) -> ()  [unwired: 1 out]
                          n266 = call <vilib>:"Digital Write Square Wave.vi"("Duration (ms)"=u32 50, "Error In"=w953, "Frequency (Hz)"=u32 365, "Channel"=u8 8, "LINX Resource"=w954) -> ("Error Out"=w945:errorcluster, "LINX Resource"=w952:T2)  [unwired: 5 in]
                          n267 = call-poly <vilib>:"Digital Write.vi"("Error In"=w945, "Output Value"=FALSE, "DO Channel"=u8 9, "LINX Resource"=w952) -> ("Error Out"=w955:errorcluster, "LINX Resource"=w956:T2)  [unwired: 6 in]
                        }
                      }
                      n268 = call "Time Delay15"("error in (no error)"=w918, "Delay Time (s)"=w902) -> ("error out"=w917:errorcluster)  [unwired: 9 in]
                      n269 = for {
                        N: 23 -> [_]
                        shift-right: [w977] -> w906
                        shift-left: w908 -> [w980]
                        shift-right: [w978] -> w907
                        shift-left: w917 -> [w979]
                        tunnel: w901 -> [w975]
                        n270 = Wait (ms)(milliseconds to wait=w975) -> ()  [unwired: 1 out]
                        n271 = for {
                          N: 30 -> [_]
                          shift-right: [w989] -> w977
                          shift-left: w980 -> [w992]
                          shift-right: [w990] -> w978
                          shift-left: w979 -> [w991]
                          n272 = Wait (ms)(milliseconds to wait=u32 40) -> ()  [unwired: 1 out]
                          n273 = call <vilib>:"Digital Write Square Wave.vi"("Duration (ms)"=u32 50, "Error In"=w991, "Frequency (Hz)"=u32 365, "Channel"=u8 6, "LINX Resource"=w992) -> ("Error Out"=w981:errorcluster, "LINX Resource"=w988:T2)  [unwired: 5 in]
                          n274 = call-poly <vilib>:"Digital Write.vi"("Error In"=w981, "Output Value"=FALSE, "DO Channel"=u8 7, "LINX Resource"=w988) -> ("Error Out"=w990:errorcluster, "LINX Resource"=w989:T2)  [unwired: 6 in]
                        }
                      }
                    }
                    n275 = local read "milliseconds to wait 2"() -> (w810:u32)
                    n276 = for {
                      N: 1 -> [_]
                      tunnel: [w833] -> w820
                      tunnel: [w832] -> w818
                      tunnel: w814 -> [w831] mode=indexing
                      tunnel: w813 -> [w830] mode=indexing
                      tunnel: w810 -> [w829]
                      n277 = Wait (ms)(milliseconds to wait=w829) -> ()  [unwired: 1 out]
                      n278 = for {
                        N: 30 -> [_]
                        tunnel: [w845] -> w833
                        tunnel: [w844] -> w832
                        tunnel: w831 -> [w843]
                        tunnel: w830 -> [w842]
                        n279 = Wait (ms)(milliseconds to wait=u32 40) -> ()  [unwired: 1 out]
                        n280 = call <vilib>:"Digital Write Square Wave.vi"("Duration (ms)"=u32 50, "Error In"=w843, "Frequency (Hz)"=u32 365, "Channel"=u8 8, "LINX Resource"=w842) -> ("Error Out"=w840:errorcluster, "LINX Resource"=w841:T2)  [unwired: 5 in]
                        n281 = call-poly <vilib>:"Digital Write.vi"("Error In"=w840, "Output Value"=FALSE, "DO Channel"=u8 9, "LINX Resource"=w841) -> ("Error Out"=w844:errorcluster, "LINX Resource"=w845:T2)  [unwired: 6 in]
                      }
                    }
                    n282 = local read "number of spots"() -> (w807:i8)
                    n283 = call "Time Delay16"("error in (no error)"=w818, "Delay Time (s)"=w807) -> ("error out"=w819:errorcluster)  [unwired: 9 in]
                    n284 = for {
                      N: 23 -> [_]
                      shift-right: [w848] -> w821
                      shift-left: w819 -> [w851]
                      shift-right: [w850] -> w816
                      shift-left: w820 -> [w849]
                      tunnel: w810 -> [w847]
                      n285 = Wait (ms)(milliseconds to wait=w847) -> ()  [unwired: 1 out]
                      n286 = for {
                        N: 30 -> [_]
                        shift-right: [w860] -> w848
                        shift-left: w851 -> [w863]
                        shift-right: [w862] -> w850
                        shift-left: w849 -> [w861]
                        n287 = Wait (ms)(milliseconds to wait=u32 40) -> ()  [unwired: 1 out]
                        n288 = call <vilib>:"Digital Write Square Wave.vi"("Duration (ms)"=u32 50, "Error In"=w863, "Frequency (Hz)"=u32 365, "Channel"=u8 6, "LINX Resource"=w861) -> ("Error Out"=w858:errorcluster, "LINX Resource"=w859:T2)  [unwired: 5 in]
                        n289 = call-poly <vilib>:"Digital Write.vi"("Error In"=w858, "Output Value"=TRUE, "DO Channel"=u8 7, "LINX Resource"=w859) -> ("Error Out"=w860:errorcluster, "LINX Resource"=w862:T2)  [unwired: 6 in]
                      }
                    }
                    n290 = call "Time Delay17"("error in (no error)"=w821, "Delay Time (s)"=w807) -> ("error out"=w822:errorcluster)  [unwired: 9 in]
                    n291 = for {
                      N: 1 -> [_]
                      shift-right: [w870] -> w815
                      shift-left: w816 -> [w868]
                      shift-right: [w869] -> w824
                      shift-left: w822 -> [w867]
                      tunnel: [w865] -> _ mode=indexing
                      tunnel: w810 -> [w864]
                      i -> [w865]
                      n292 = Wait (ms)(milliseconds to wait=w864) -> ()  [unwired: 1 out]
                      n293 = for {
                        N: 30 -> [_]
                        shift-right: [w882] -> w870
                        shift-left: w868 -> [w880]
                        shift-right: [w881] -> w869
                        shift-left: w867 -> [w879]
                        n294 = Wait (ms)(milliseconds to wait=u32 40) -> ()  [unwired: 1 out]
                        n295 = call <vilib>:"Digital Write Square Wave.vi"("Duration (ms)"=u32 50, "Error In"=w879, "Frequency (Hz)"=u32 365, "Channel"=u8 8, "LINX Resource"=w880) -> ("Error Out"=w871:errorcluster, "LINX Resource"=w878:T2)  [unwired: 5 in]
                        n296 = call-poly <vilib>:"Digital Write.vi"("Error In"=w871, "Output Value"=FALSE, "DO Channel"=u8 9, "LINX Resource"=w878) -> ("Error Out"=w881:errorcluster, "LINX Resource"=w882:T2)  [unwired: 6 in]
                      }
                    }
                    n297 = call "Time Delay18"("error in (no error)"=w824, "Delay Time (s)"=w807) -> ("error out"=w823:errorcluster)  [unwired: 9 in]
                    n298 = local read "R of B/49"() -> (w805:dbl)
                    n299 = for {
                      N: w805 -> [_]
                      shift-right: [w885] -> w811
                      shift-left: w815 -> [w888]
                      shift-right: [w886] -> w809
                      shift-left: w823 -> [w887]
                      tunnel: w810 -> [w883]
                      n300 = Wait (ms)(milliseconds to wait=w883) -> ()  [unwired: 1 out]
                      n301 = for {
                        N: 30 -> [_]
                        shift-right: [w897] -> w885
                        shift-left: w888 -> [w900]
                        shift-right: [w898] -> w886
                        shift-left: w887 -> [w899]
                        n302 = Wait (ms)(milliseconds to wait=u32 40) -> ()  [unwired: 1 out]
                        n303 = call <vilib>:"Digital Write Square Wave.vi"("Duration (ms)"=u32 50, "Error In"=w899, "Frequency (Hz)"=u32 365, "Channel"=u8 6, "LINX Resource"=w900) -> ("Error Out"=w889:errorcluster, "LINX Resource"=w896:T2)  [unwired: 5 in]
                        n304 = call-poly <vilib>:"Digital Write.vi"("Error In"=w889, "Output Value"=TRUE, "DO Channel"=u8 7, "LINX Resource"=w896) -> ("Error Out"=w898:errorcluster, "LINX Resource"=w897:T2)  [unwired: 6 in]
                      }
                    }
                    n305 = call "Time Delay20"("error in (no error)"=w809, "Delay Time (s)"=w807) -> ("error out"=w808:errorcluster)  [unwired: 9 in]
                  }
                }
              }
              frame True {
                # "Second case True"
                n306 = local read "R of B/49"() -> (w995:dbl)
                n307 = case shown="25..48" w995 {
                  tunnel: w997 -> [w1001 w1025 w1073 w1143]
                  tunnel: w996 -> [w1000 w1024 w1072 w1142]
                  tunnel: [w999 w1027 w1074 w1144] -> w994
                  tunnel: [w998 w1026 w1075 w1145] -> w993
                  frame 1, Default {
                    # "Go down 1 step"
                    # "Third case"
                    n308 = local read "milliseconds to wait 2"() -> (w1002:u32)
                    n309 = for {
                      N: 1 -> [_]
                      shift-right: [w1010] -> w998
                      shift-left: w1001 -> [w1009]
                      shift-right: [w1011] -> w1003
                      shift-left: w1000 -> [w1008]
                      tunnel: w1002 -> [w1006]
                      n310 = Wait (ms)(milliseconds to wait=w1006) -> ()  [unwired: 1 out]
                      n311 = for {
                        N: 30 -> [_]
                        shift-right: [w1022] -> w1010
                        shift-left: w1009 -> [w1021]
                        shift-right: [w1023] -> w1011
                        shift-left: w1008 -> [w1020]
                        n312 = Wait (ms)(milliseconds to wait=u32 40) -> ()  [unwired: 1 out]
                        n313 = call <vilib>:"Digital Write Square Wave.vi"("Duration (ms)"=u32 50, "Error In"=w1020, "Frequency (Hz)"=u32 365, "Channel"=u8 8, "LINX Resource"=w1021) -> ("Error Out"=w1018:errorcluster, "LINX Resource"=w1019:T2)  [unwired: 5 in]
                        n314 = call-poly <vilib>:"Digital Write.vi"("Error In"=w1018, "Output Value"=FALSE, "DO Channel"=u8 9, "LINX Resource"=w1019) -> ("Error Out"=w1023:errorcluster, "LINX Resource"=w1022:T2)  [unwired: 6 in]
                      }
                    }
                    n315 = local read "number of spots"() -> (w1004:i8)
                    n316 = call "Time Delay7"("error in (no error)"=w1003, "Delay Time (s)"=w1004) -> ("error out"=w999:errorcluster)  [unwired: 9 in]
                  }
                  frame 2..23 {
                    # "Go left 23 steps"
                    # "Go down 1 step"
                    # "Third case True"
                    n317 = local read "milliseconds to wait 2"() -> (w1031:u32)
                    n318 = for {
                      N: 1 -> [_]
                      shift-right: [w1058] -> w1032
                      shift-left: w1025 -> [w1057]
                      shift-right: [w1059] -> w1034
                      shift-left: w1024 -> [w1056]
                      tunnel: w1031 -> [w1054]
                      n319 = Wait (ms)(milliseconds to wait=w1054) -> ()  [unwired: 1 out]
                      n320 = for {
                        N: 30 -> [_]
                        shift-right: [w1070] -> w1058
                        shift-left: w1057 -> [w1069]
                        shift-right: [w1071] -> w1059
                        shift-left: w1056 -> [w1068]
                        n321 = Wait (ms)(milliseconds to wait=u32 40) -> ()  [unwired: 1 out]
                        n322 = call <vilib>:"Digital Write Square Wave.vi"("Duration (ms)"=u32 50, "Error In"=w1068, "Frequency (Hz)"=u32 365, "Channel"=u8 8, "LINX Resource"=w1069) -> ("Error Out"=w1066:errorcluster, "LINX Resource"=w1067:T2)  [unwired: 5 in]
                        n323 = call-poly <vilib>:"Digital Write.vi"("Error In"=w1066, "Output Value"=FALSE, "DO Channel"=u8 9, "LINX Resource"=w1067) -> ("Error Out"=w1071:errorcluster, "LINX Resource"=w1070:T2)  [unwired: 6 in]
                      }
                    }
                    n324 = local read "B-1\n= # of spots in the last row\n= (# of spots - first row -1)"() -> (w1028:dbl)
                    n325 = local read "number of spots"() -> (w1029:i8)
                    n326 = call "Time Delay5"("error in (no error)"=w1034, "Delay Time (s)"=w1029) -> ("error out"=w1033:errorcluster)  [unwired: 9 in]
                    n327 = for {
                      N: w1028 -> [_]
                      shift-right: [w1038] -> w1030
                      shift-left: w1033 -> [w1041]
                      shift-right: [w1040] -> w1026
                      shift-left: w1032 -> [w1039]
                      tunnel: w1031 -> [w1036]
                      n328 = Wait (ms)(milliseconds to wait=w1036) -> ()  [unwired: 1 out]
                      n329 = for {
                        N: 30 -> [_]
                        shift-right: [w1050] -> w1038
                        shift-left: w1041 -> [w1053]
                        shift-right: [w1052] -> w1040
                        shift-left: w1039 -> [w1051]
                        n330 = Wait (ms)(milliseconds to wait=u32 40) -> ()  [unwired: 1 out]
                        n331 = call <vilib>:"Digital Write Square Wave.vi"("Duration (ms)"=u32 50, "Error In"=w1053, "Frequency (Hz)"=u32 365, "Channel"=u8 6, "LINX Resource"=w1051) -> ("Error Out"=w1048:errorcluster, "LINX Resource"=w1049:T2)  [unwired: 5 in]
                        n332 = call-poly <vilib>:"Digital Write.vi"("Error In"=w1048, "Output Value"=FALSE, "DO Channel"=u8 7, "LINX Resource"=w1049) -> ("Error Out"=w1050:errorcluster, "LINX Resource"=w1052:T2)  [unwired: 6 in]
                      }
                    }
                    n333 = call "Time Delay6"("error in (no error)"=w1030, "Delay Time (s)"=w1029) -> ("error out"=w1027:errorcluster)  [unwired: 9 in]
                  }
                  frame 24 {
                    # "Go right 23 step"
                    # "Go down 1 step"
                    # "Go left 23 steps"
                    # "Go down 1 step"
                    n334 = local read "milliseconds to wait 2"() -> (w1087:u32)
                    n335 = for {
                      N: 1 -> [_]
                      shift-right: [w1128] -> w1083
                      shift-left: w1073 -> [w1127]
                      shift-right: [w1129] -> w1081
                      shift-left: w1072 -> [w1126]
                      tunnel: w1087 -> [w1124]
                      n336 = Wait (ms)(milliseconds to wait=w1124) -> ()  [unwired: 1 out]
                      n337 = for {
                        N: 30 -> [_]
                        shift-right: [w1140] -> w1128
                        shift-left: w1127 -> [w1139]
                        shift-right: [w1141] -> w1129
                        shift-left: w1126 -> [w1138]
                        n338 = Wait (ms)(milliseconds to wait=u32 40) -> ()  [unwired: 1 out]
                        n339 = call <vilib>:"Digital Write Square Wave.vi"("Duration (ms)"=u32 50, "Error In"=w1138, "Frequency (Hz)"=u32 365, "Channel"=u8 8, "LINX Resource"=w1139) -> ("Error Out"=w1136:errorcluster, "LINX Resource"=w1137:T2)  [unwired: 5 in]
                        n340 = call-poly <vilib>:"Digital Write.vi"("Error In"=w1136, "Output Value"=FALSE, "DO Channel"=u8 9, "LINX Resource"=w1137) -> ("Error Out"=w1141:errorcluster, "LINX Resource"=w1140:T2)  [unwired: 6 in]
                      }
                    }
                    n341 = local read "number of spots"() -> (w1076:i8)
                    n342 = call "Time Delay21"("error in (no error)"=w1081, "Delay Time (s)"=w1076) -> ("error out"=w1082:errorcluster)  [unwired: 9 in]
                    n343 = for {
                      N: 23 -> [_]
                      shift-right: [w1090] -> w1084
                      shift-left: w1082 -> [w1093]
                      shift-right: [w1092] -> w1078
                      shift-left: w1083 -> [w1091]
                      tunnel: w1087 -> [w1089]
                      n344 = Wait (ms)(milliseconds to wait=w1089) -> ()  [unwired: 1 out]
                      n345 = for {
                        N: 30 -> [_]
                        shift-right: [w1102] -> w1090
                        shift-left: w1093 -> [w1105]
                        shift-right: [w1104] -> w1092
                        shift-left: w1091 -> [w1103]
                        n346 = Wait (ms)(milliseconds to wait=u32 40) -> ()  [unwired: 1 out]
                        n347 = call <vilib>:"Digital Write Square Wave.vi"("Duration (ms)"=u32 50, "Error In"=w1105, "Frequency (Hz)"=u32 365, "Channel"=u8 6, "LINX Resource"=w1103) -> ("Error Out"=w1100:errorcluster, "LINX Resource"=w1101:T2)  [unwired: 5 in]
                        n348 = call-poly <vilib>:"Digital Write.vi"("Error In"=w1100, "Output Value"=FALSE, "DO Channel"=u8 7, "LINX Resource"=w1101) -> ("Error Out"=w1102:errorcluster, "LINX Resource"=w1104:T2)  [unwired: 6 in]
                      }
                    }
                    n349 = call "Time Delay22"("error in (no error)"=w1084, "Delay Time (s)"=w1076) -> ("error out"=w1085:errorcluster)  [unwired: 9 in]
                    n350 = for {
                      N: 1 -> [_]
                      shift-right: [w1111] -> w1075
                      shift-left: w1078 -> [w1109]
                      shift-right: [w1110] -> w1077
                      shift-left: w1085 -> [w1108]
                      tunnel: w1087 -> [w1106]
                      n351 = Wait (ms)(milliseconds to wait=w1106) -> ()  [unwired: 1 out]
                      n352 = for {
                        N: 30 -> [_]
                        shift-right: [w1123] -> w1111
                        shift-left: w1109 -> [w1121]
                        shift-right: [w1122] -> w1110
                        shift-left: w1108 -> [w1120]
                        n353 = Wait (ms)(milliseconds to wait=u32 40) -> ()  [unwired: 1 out]
                        n354 = call <vilib>:"Digital Write Square Wave.vi"("Duration (ms)"=u32 50, "Error In"=w1120, "Frequency (Hz)"=u32 365, "Channel"=u8 8, "LINX Resource"=w1121) -> ("Error Out"=w1112:errorcluster, "LINX Resource"=w1119:T2)  [unwired: 5 in]
                        n355 = call-poly <vilib>:"Digital Write.vi"("Error In"=w1112, "Output Value"=FALSE, "DO Channel"=u8 9, "LINX Resource"=w1119) -> ("Error Out"=w1122:errorcluster, "LINX Resource"=w1123:T2)  [unwired: 6 in]
                      }
                    }
                    n356 = call "Time Delay8"("error in (no error)"=w1077, "Delay Time (s)"=w1076) -> ("error out"=w1074:errorcluster)  [unwired: 9 in]
                  }
                  frame 25..48 {
                    # "move away from the y motor B-25 steps"
                    # "move to the y motor 23 steps"
                    # "move away from the x motor 1 step"
                    n357 = local read "milliseconds to wait 2"() -> (w1148:u32)
                    n358 = for {
                      N: 1 -> [_]
                      shift-right: [w1203] -> w1152
                      shift-left: w1143 -> [w1202]
                      shift-right: [w1204] -> w1154
                      shift-left: w1142 -> [w1201]
                      tunnel: w1148 -> [w1199]
                      n359 = Wait (ms)(milliseconds to wait=w1199) -> ()  [unwired: 1 out]
                      n360 = for {
                        N: 30 -> [_]
                        shift-right: [w1215] -> w1203
                        shift-left: w1202 -> [w1214]
                        shift-right: [w1216] -> w1204
                        shift-left: w1201 -> [w1213]
                        n361 = Wait (ms)(milliseconds to wait=u32 40) -> ()  [unwired: 1 out]
                        n362 = call <vilib>:"Digital Write Square Wave.vi"("Duration (ms)"=u32 50, "Error In"=w1213, "Frequency (Hz)"=u32 365, "Channel"=u8 8, "LINX Resource"=w1214) -> ("Error Out"=w1211:errorcluster, "LINX Resource"=w1212:T2)  [unwired: 5 in]
                        n363 = call-poly <vilib>:"Digital Write.vi"("Error In"=w1211, "Output Value"=FALSE, "DO Channel"=u8 9, "LINX Resource"=w1212) -> ("Error Out"=w1216:errorcluster, "LINX Resource"=w1215:T2)  [unwired: 6 in]
                      }
                    }
                    n364 = local read "Time per spots(s)"() -> (w1146:i8)
                    n365 = call "Time Delay24"("error in (no error)"=w1154, "Delay Time (s)"=w1146) -> ("error out"=w1153:errorcluster)  [unwired: 9 in]
                    n366 = for {
                      N: 23 -> [_]
                      shift-right: [w1164] -> w1151
                      shift-left: w1153 -> [w1167]
                      shift-right: [w1166] -> w1157
                      shift-left: w1152 -> [w1165]
                      tunnel: w1148 -> [w1163]
                      n367 = Wait (ms)(milliseconds to wait=w1163) -> ()  [unwired: 1 out]
                      n368 = for {
                        N: 30 -> [_]
                        shift-right: [w1176] -> w1164
                        shift-left: w1167 -> [w1179]
                        shift-right: [w1178] -> w1166
                        shift-left: w1165 -> [w1177]
                        n369 = Wait (ms)(milliseconds to wait=u32 40) -> ()  [unwired: 1 out]
                        n370 = call <vilib>:"Digital Write Square Wave.vi"("Duration (ms)"=u32 50, "Error In"=w1179, "Frequency (Hz)"=u32 365, "Channel"=u8 6, "LINX Resource"=w1177) -> ("Error Out"=w1174:errorcluster, "LINX Resource"=w1175:T2)  [unwired: 5 in]
                        n371 = call-poly <vilib>:"Digital Write.vi"("Error In"=w1174, "Output Value"=TRUE, "DO Channel"=u8 7, "LINX Resource"=w1175) -> ("Error Out"=w1176:errorcluster, "LINX Resource"=w1178:T2)  [unwired: 6 in]
                      }
                    }
                    n372 = call "Time Delay25"("error in (no error)"=w1151, "Delay Time (s)"=w1146) -> ("error out"=w1150:errorcluster)  [unwired: 9 in]
                    n373 = for {
                      N: 1 -> [_]
                      shift-right: [w1186] -> w1161
                      shift-left: w1157 -> [w1184]
                      shift-right: [w1185] -> w1159
                      shift-left: w1150 -> [w1183]
                      tunnel: [w1181] -> _ mode=indexing
                      tunnel: w1148 -> [w1180]
                      i -> [w1181]
                      # "move away from the x motor 1 step"
                      n374 = Wait (ms)(milliseconds to wait=w1180) -> ()  [unwired: 1 out]
                      n375 = for {
                        N: 30 -> [_]
                        shift-right: [w1198] -> w1186
                        shift-left: w1184 -> [w1196]
                        shift-right: [w1197] -> w1185
                        shift-left: w1183 -> [w1195]
                        n376 = Wait (ms)(milliseconds to wait=u32 40) -> ()  [unwired: 1 out]
                        n377 = call <vilib>:"Digital Write Square Wave.vi"("Duration (ms)"=u32 50, "Error In"=w1195, "Frequency (Hz)"=u32 365, "Channel"=u8 8, "LINX Resource"=w1196) -> ("Error Out"=w1187:errorcluster, "LINX Resource"=w1194:T2)  [unwired: 5 in]
                        n378 = call-poly <vilib>:"Digital Write.vi"("Error In"=w1187, "Output Value"=FALSE, "DO Channel"=u8 9, "LINX Resource"=w1194) -> ("Error Out"=w1197:errorcluster, "LINX Resource"=w1198:T2)  [unwired: 6 in]
                      }
                    }
                    n379 = local read "milliseconds to wait 2"() -> (w1158:u32)
                    n380 = call "Time Delay23"("error in (no error)"=w1159, "Delay Time (s)"=w1146) -> ("error out"=w1160:errorcluster)  [unwired: 9 in]
                    n381 = local read "B-25"() -> (w1147:dbl)
                    n382 = for {
                      N: w1147 -> [_]
                      shift-right: [w1219] -> w1145
                      shift-left: w1161 -> [w1222]
                      shift-right: [w1220] -> w1144
                      shift-left: w1160 -> [w1221]
                      tunnel: w1158 -> [w1217]
                      n383 = Wait (ms)(milliseconds to wait=w1217) -> ()  [unwired: 1 out]
                      n384 = for {
                        N: 30 -> [_]
                        shift-right: [w1231] -> w1219
                        shift-left: w1222 -> [w1234]
                        shift-right: [w1232] -> w1220
                        shift-left: w1221 -> [w1233]
                        n385 = Wait (ms)(milliseconds to wait=u32 40) -> ()  [unwired: 1 out]
                        n386 = call <vilib>:"Digital Write Square Wave.vi"("Duration (ms)"=u32 50, "Error In"=w1233, "Frequency (Hz)"=u32 365, "Channel"=u8 6, "LINX Resource"=w1234) -> ("Error Out"=w1223:errorcluster, "LINX Resource"=w1230:T2)  [unwired: 5 in]
                        n387 = call-poly <vilib>:"Digital Write.vi"("Error In"=w1223, "Output Value"=FALSE, "DO Channel"=u8 7, "LINX Resource"=w1230) -> ("Error Out"=w1232:errorcluster, "LINX Resource"=w1231:T2)  [unwired: 6 in]
                      }
                    }
                  }
                }
              }
            }
          }
          frame True {
            # "First case Ture"
            n388 = local read "Last point(column)-Start point(column)"() -> (w1253:dbl)
            n389 = for {
              N: w1253 -> [_]
              shift-right: [w1261] -> w1255
              shift-left: w1257 -> [w1263]
              shift-right: [w1260] -> w1254
              shift-left: w1256 -> [w1262]
              n390 = for {
                N: 30 -> [_]
                shift-right: [w1273] -> w1261
                shift-left: w1263 -> [w1275]
                shift-right: [w1272] -> w1260
                shift-left: w1262 -> [w1274]
                n391 = Wait (ms)(milliseconds to wait=u32 40) -> ()  [unwired: 1 out]
                n392 = call <vilib>:"Digital Write Square Wave.vi"("Duration (ms)"=u32 50, "Error In"=w1274, "Frequency (Hz)"=u32 365, "Channel"=u8 6, "LINX Resource"=w1275) -> ("Error Out"=w1270:errorcluster, "LINX Resource"=w1271:T2)  [unwired: 5 in]
                n393 = call-poly <vilib>:"Digital Write.vi"("Error In"=w1270, "Output Value"=FALSE, "DO Channel"=u8 7, "LINX Resource"=w1271) -> ("Error Out"=w1272:errorcluster, "LINX Resource"=w1273:T2)  [unwired: 6 in]
              }
              n394 = local read "milliseconds to wait 2"() -> (w1258:u32)
              n395 = Wait (ms)(milliseconds to wait=w1258) -> ()  [unwired: 1 out]
            }
          }
        }
        n396 = Equal?(x=w166, y=0.0) -> (x = y?=→"IQ of B/49 = 0":bool)
        n397 = Quotient & Remainder(x=w172, y=25.0) -> (x-y*floor(x/y)=w151:dbl, floor(x/y)=w170:dbl)
        n398 = Equal?(x=w170, y=0.0) -> (x = y?=→"IQ of B/25 = 0":bool)
        n399 = Subtract(x=w151, y=25.0) -> (x-y=→"B-25":dbl)
        n400 = while {
          tunnel: [w266] -> w188
          tunnel: [w267] -> w187
          tunnel: w178 -> [w260]
          tunnel: w177 -> [w259]
          stop <- w262 stop-if-true
          n401 = Wait (ms)(milliseconds to wait=u32 40) -> ()  [unwired: 1 out]
          n402 = call <vilib>:"Digital Write Square Wave.vi"("Duration (ms)"=u32 50, "Error In"=w260, "Frequency (Hz)"=u32 450, "Channel"=u8 8, "LINX Resource"=w259) -> ("Error Out"=w261:errorcluster, "LINX Resource"=w274:T2)  [unwired: 5 in]
          n403 = call-poly <vilib>:"Digital Write.vi"("Error In"=w261, "Output Value"=TRUE, "DO Channel"=u8 9, "LINX Resource"=w274) -> ("Error Out"=w264:errorcluster, "LINX Resource"=w265:T2)  [unwired: 6 in]
          n404 = call-poly <vilib>:"Digital Read.vi"("Error In"=w264, "DI Channel"=u8 5 ("Analog Channel"), "LINX Resource"=w265) -> ("Error Out"=w267:errorcluster, "DI Value"=w262:bool, "LINX Resource"=w266:T2)  [unwired: 6 in]
        }
        n405 = for {
          N: 250 -> [_]
          tunnel: w188 -> [w251]
          tunnel: [w248] -> w185
          tunnel: [w249] -> w184
          tunnel: w187 -> [w244]
          n406 = Wait (ms)(milliseconds to wait=u32 40) -> ()  [unwired: 1 out]
          n407 = call <vilib>:"Digital Write Square Wave.vi"("Duration (ms)"=u32 50, "Error In"=w244, "Frequency (Hz)"=u32 450, "Channel"=u8 8, "LINX Resource"=w251) -> ("Error Out"=w257:errorcluster, "LINX Resource"=w258:T2)  [unwired: 5 in]
          n408 = call-poly <vilib>:"Digital Write.vi"("Error In"=w257, "Output Value"=FALSE, "DO Channel"=u8 9, "LINX Resource"=w258) -> ("Error Out"=w246:errorcluster, "LINX Resource"=w247:T2)  [unwired: 6 in]
          n409 = call-poly <vilib>:"Digital Read.vi"("Error In"=w246, "DI Channel"=u8 5 ("Analog Channel"), "LINX Resource"=w247) -> ("Error Out"=w249:errorcluster, "LINX Resource"=w248:T2)  [unwired: 6 in, 1 out]
        }
        n410 = while {
          tunnel: [w231] -> w183
          shift-right: [w229] -> w182
          shift-left: w184 -> [w243]
          tunnel: w185 -> [w235]
          stop <- w228 stop-if-true
          n411 = Wait (ms)(milliseconds to wait=u32 40) -> ()  [unwired: 1 out]
          n412 = call <vilib>:"Digital Write Square Wave.vi"("Duration (ms)"=u32 50, "Error In"=w243, "Frequency (Hz)"=u32 450, "Channel"=u8 6, "LINX Resource"=w235) -> ("Error Out"=w241:errorcluster, "LINX Resource"=w242:T2)  [unwired: 5 in]
          n413 = call-poly <vilib>:"Digital Write.vi"("Error In"=w241, "Output Value"=TRUE, "DO Channel"=u8 7, "LINX Resource"=w242) -> ("Error Out"=w230:errorcluster, "LINX Resource"=w232:T2)  [unwired: 6 in]
          n414 = call-poly <vilib>:"Digital Read.vi"("Error In"=w230, "DI Channel"=u8 4 ("Analog Channel"), "LINX Resource"=w232) -> ("Error Out"=w229:errorcluster, "DI Value"=w228:bool, "LINX Resource"=w231:T2)  [unwired: 6 in]
        }
        n415 = for {
          N: 250 -> [_]
          tunnel: [w215] -> w180
          shift-right: [w213] -> w179
          shift-left: w182 -> [w227]
          tunnel: w183 -> [w219]
          n416 = Wait (ms)(milliseconds to wait=u32 40) -> ()  [unwired: 1 out]
          n417 = call <vilib>:"Digital Write Square Wave.vi"("Duration (ms)"=u32 50, "Error In"=w227, "Frequency (Hz)"=u32 450, "Channel"=u8 6, "LINX Resource"=w219) -> ("Error Out"=w225:errorcluster, "LINX Resource"=w226:T2)  [unwired: 5 in]
          n418 = call-poly <vilib>:"Digital Write.vi"("Error In"=w225, "Output Value"=FALSE, "DO Channel"=u8 7, "LINX Resource"=w226) -> ("Error Out"=w214:errorcluster, "LINX Resource"=w216:T2)  [unwired: 6 in]
          n419 = call-poly <vilib>:"Digital Read.vi"("Error In"=w214, "DI Channel"=u8 4 ("Analog Channel"), "LINX Resource"=w216) -> ("Error Out"=w213:errorcluster, "LINX Resource"=w215:T2)  [unwired: 6 in, 1 out]
        }
      }
    }
  }
  n420 = call <vilib>:"Close.vi"("Error In"=w1, "LINX Resource"=w2) -> ("Error Out"=w5:errorcluster)  [unwired: 9 in]
  n421 = call <vilib>:"Simple Error Handler.vi"("error in (no error)"=w5) -> ()  [unwired: 4 in, 5 out]
